vi "pco.labview_Example.vi"() -> ()   [LabVIEW 2020]
uses:
  CameraAccess.lvlib
  Structures.lvlib
  RecordingControl.lvlib
  ImageSensor.lvlib
  GeneralCameraControl.lvlib
  Recorder.lvlib
  TimingControl.lvlib
panel:
  out "exposureMinLimit":u64
  out "exposureMaxLimit":u64
  out "strSensor":T1
  in  "wRegionType":u16(ring) items=["REGION_TYPE_BALANCED", "REGION_TYPE_CENTER_BASED", "REGION_TYPE_CORNER_BASED", "REGION_TYPE_FULL", "REGION_TYPE_CUSTOM"]
  in  "wExpBase":u16(ring)=2 items=["ns", "us", "ms"]
  in  "dwMinExposure":u32=1 min=1 step=1
  in  "dwMaxExposure":u32=100 min=1 step=1
  in  "wSmoothness":u16=1 caption="Smoothness" min=1 max=10 step=1
  in  "bAutoExp":bool caption="Auto Exp On"
  in  "wRamSegment":u16[](array[numeric]) caption="Ram Segment\n(only CamRam)"
  in  "Get Image":bool
  out "bFIFOOverflow":bool[](array[boolean]) caption="FIFO Overflow"
  in  "Init":bool
  in  "baseName":string caption="Base File Name \n(only file, not mandatory)"
  in  "ResetRecorder":bool caption="Stop Copy"
  out "Image":u16[][](graph)
  in  "Quit":bool
  in  "Stop recording":bool
  in  "Start recording":bool
  in  "Create":bool
  in  "roiY1":u16=2 min=2 max=5120 step=1
  in  "roiX1":u16=2 min=2 max=896 step=1
  in  "roiY0":u16=1 min=1 max=5119 step=1
  in  "roiX0":u16=1 min=1 max=895 step=1
  out "Image Height":u16
  out "Image Width":u16
  in  "Image Index":u32 max=9
  in  "Cam Index":u32 max=0 step=1
  out "dwReqImgCount":u32[](array[numeric]) caption="Required Number of Images (Indicator)"
  out "stopTime[ms]":u32[](array[numeric]) caption="Stop Time  of Record [ms]"
  out "bBuffersFull":bool[](array[boolean]) caption="ReqImg Recorded"
  out "dwProcImgCount":u32[](array[numeric]) caption="Currently Recorded Images"
  out "lastError":u32[](array[numeric]) caption="Last Error" format="%x"
  out "bIsRunning":bool[](array[boolean]) caption="Acquiring Flag"
  out "startTime[ms]":u32[](array[numeric]) caption="Start Time  of Record [ms]"
  in  "dwImgCountArr":u32[](array[numeric]) caption="Required Number \nof Images" min=4
  out "phRec":u64
  out "dwMaxImgCountArr":u32[](array[numeric]) caption="Max Number of Recordable Images"
  in  "dwImgDistributionArr":u32[](array[numeric]) caption="Memory Distribution" min=1
  in  "szPath":path=path "C:/" caption="Destination Folder"
  in  "wType":u16(ring)=1 caption="Type" items=["PCO_RECORDER_MEMORY_SEQUENCE"=1, "PCO_RECORDER_MEMORY_RINGBUF"=2, "PCO_RECORDER_MEMORY_FIFO"=3]
  in  "dwRecMode":u16(ring)=1 caption="Recorder Mode" items=["PCO_RECORDER_MODE_FILE"=1, "PCO_RECORDER_MODE_MEMORY"=2, "PCO_RECORDER_MODE_CAMRAM"=3]
  out "Error":errorcluster {"code" format="%x"}
  out "phCam":u64[](array[numeric])
  # "This is the main example program showing the different possibilities of recording images with pco cameras\nThe usage is guided by disabling/enabling the required parts of the front panel.\nLive images are shown during record\nImages can be read after acquisition is finished/stopped\nFor detailed information watch the Use_pco.labview_Example.avi video\n\n+ If you want a example with live stream images, take a look at pco.labview_Live_Example.vi\n+ If you want a small example to start building your own application, you can also use pco.labview_Simple_example.vi"
  # "pco.labview"
  # "Create Parameters"
  # "Auto Exposure"
  # "Init Parameters"
  # "Acquire Images"
  # "Status Indicators"
  # "Parameters for image readout"
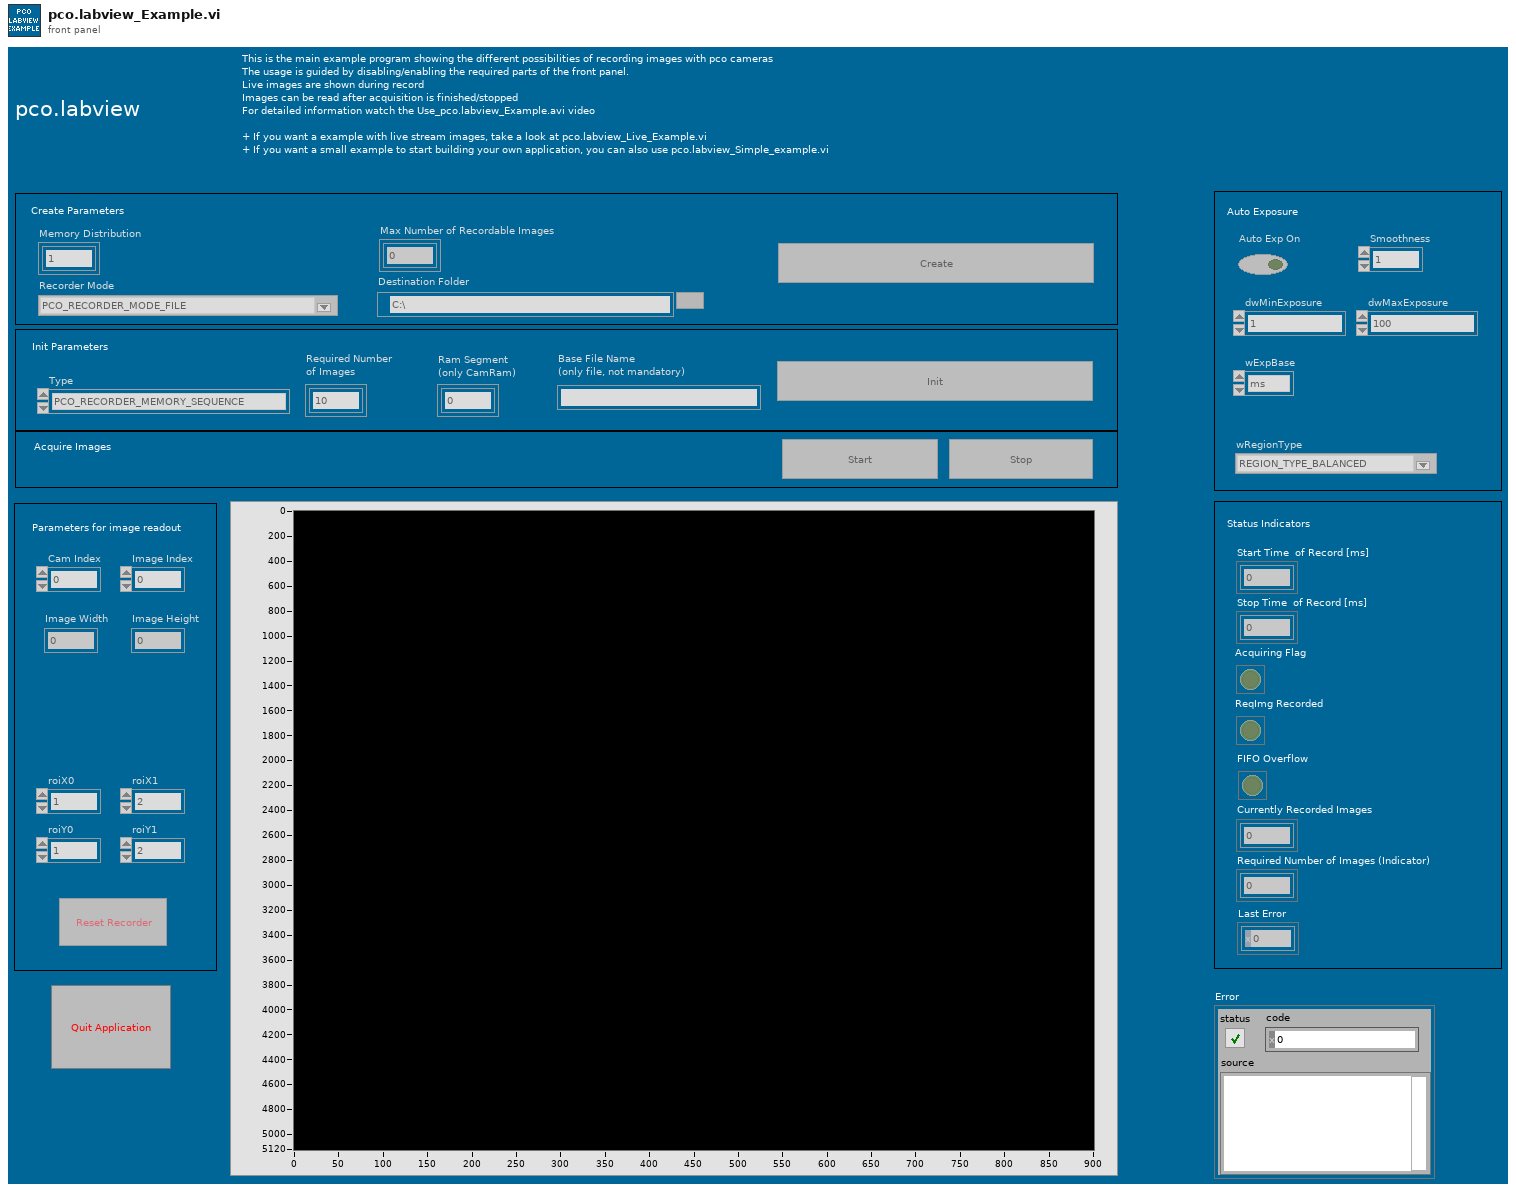
[diagram p1: front panel]
types:
  T1 = cluster{"PCO_Description":cluster{"wSensorTypeDESC":u16, "wSensorSubTypeDESC":u16, "wMaxHorzResStdDESC":u16, "wMaxVertResStdDESC":u16, "wMaxHorzResExtDESC":u16, "wMaxVertResExtDESC":u16, "wDynResDESC":u16, "wMaxBinHorzDESC":u16, "wBinHorzSteppingDESC":u16, "wMaxBinVertDESC":u16, "wBinVertSteppingDESC":u16, "wRoiHorStepsDESC":u16, "wRoiVertStepsDESC":u16, "wNumADCsDESC":u16, "wMinSizeHorzDESC":u16, "dwPixelRateDESC":u32[], "wConvFactDESC":u16[], "sCoolingSetpoints":i16[], "wSoftRoiHorStepsDESC":u16, "wSoftRoiVertStepsDESC":u16, "wIRDESC":u16, "wMinSizeVertDESC":u16, "dwMinDelayDESC":u32, "dwMaxDelayDESC":u32, "dwMinDelayStepDESC":u32, "dwMinExposureDESC":u32, "dwMaxExposureDESC":u32, "dwMinExposureStepDESC":u32, "dwMinDelayIRDESC":u32, "dwMaxDelayIRDESC":u32, "dwMinExposureIRDESC":u32, "dwMaxExposureIRDESC":u32, "wTimeTableDESC":u16, "wDoubleImageDESC":u16, "sMinCoolSetDESC":i16, "sMaxCoolSetDESC":i16, "sDefaultCoolSetDESC":i16, "wPowerDownModeDESC":u16, "wOffsetRegulationDESC":u16, "wColorPatternDESC":u16, "wPatternTypeDESC":u16, "wNumCoolingSetpoints":u16, "dwGeneralCapsDESC1":u32, "dwGeneralCapsDESC2":u32, "dwExtSyncFrequency":u32[], "dwGeneralCapsDESC3":u32, "dwGeneralCapsDESC4":u32}, "PCO_Description2":cluster{"dwMinPeriodicalTimeDESC2":u32, "dwMaxPeriodicalTimeDESC2":u32, "dwMinPeriodicalConditionDESC2":u32, "dwMaxNumberOfExposuresDESC2":u32, "lMinMonitorSignalOffsetDESC2":i32, "dwMaxMonitorSignalOffsetDESC2":u32, "dwMinPeriodicalStepDESC2":u32, "dwStartTimeDelayDESC2":u32, "dwMinMonitorStepDESC2":u32, "dwMinDelayModDESC2":u32, "dwMaxDelayModDESC2":u32, "dwMinDelayStepModDESC2":u32, "dwMinExposureModDESC2":u32, "dwMaxExposureModDESC2":u32, "dwMinExposureStepModDESC2":u32, "dwModulateCapsDESC2":u32}, "PCO_Description_Intensified":cluster{"wChannelNumberIntensifiedDESC":u16, "wNumberOfChannelsIntensifiedDESC":u16, "wMinVoltageIntensifiedDESC":u16, "wMaxVoltageIntensifiedDESC":u16, "wVoltageStepIntensifiedDESC":u16, "wExtendedMinVoltageIntensifiedDESC":u16, "wMaxLoopCountIntensifiedDESC":u16, "dwMinPhosphorDecayIntensified_ns_DESC":u32, "dwMaxPhosphorDecayIntensified_ms_DESC":u32, "dwFlagsIntensifiedDESC":u32, "szIntensifierTypeDESC":string, "dwMCP_RectangleXL_DESC":u32, "dwMCP_RectangleXR_DESC":u32, "dwMCP_RectangleYT_DESC":u32, "dwMCP_RectangleYB_DESC":u32}, "PCO_Description3":cluster{"wDarkOffsetDESC3":u16, "dwGeneralCapsDESC3_1":u32, "dwGeneralCapsDESC3_2":u32, "dwGeneralCapsDESC3_3":u32, "dwGeneralCapsDESC3_4":u32, "wMinHorzResStdDESC3":u16, "wMinVertResStdDESC3":u16, "wMinHorzResExtDESC3":u16, "wMinVertResExtDESC3":u16, "dPixelsize_horzDESC3_um":dbl, "dPixelsize_vertDESC3_um":dbl, "dMinSensorTempWarningDESC3_C":dbl, "dMaxSensorTempWarningDESC3_C":dbl, "dMinCameraTempWarningDESC3_C":dbl, "dMaxCameraTempWarningDESC3_C":dbl, "dMinPowerTempWarningDESC3_C":dbl, "dMaxPowerTempWarningDESC3_C":dbl, "dMinPowerVoltageWarningDESC3_V":dbl, "dMaxPowerVoltageWarningDESC3_V":dbl, "dMinSensorTempErrorDESC3_C":dbl, "dMaxSensorTempErrorDESC3_C":dbl, "dMinCameraTempErrorDESC3_C":dbl, "dMaxCameraTempErrorDESC3_C":dbl, "dMinPowerTempErrorDESC3_C":dbl, "dMaxPowerTempErrorDESC3_C":dbl, "dMinPowerVoltageErrorDESC3_V":dbl, "dMaxPowerVoltageErrorDESC3_V":dbl}, "wSensorformat":u16, "wRoiX0":u16, "wRoiY0":u16, "wRoiX1":u16, "wRoiY1":u16, "wBinHorz":u16, "wBinVert":u16, "wIntensifiedFlags":u16, "dwPixelRate":u32, "wConvFact":u16, "wDoubleImage":u16, "wADCOperation":u16, "wIR":u16, "sCoolSet":i16, "wOffsetRegulation":u16, "wNoiseFilterMode":u16, "wFastReadoutMode":u16, "wDSNUAdjustMode":u16, "wCDIMode":u16, "wIntensifiedVoltage":u16, "wIntensifiedGatingMode":u16, "dwIntensifiedPhosphorDecay_us":u32, "PCO_Signal_Description":cluster{"wNumOfSignals":u16, "strSingeSignalDesc":cluster{"strSignalName":string[], "wSignalDefinitions":u16, "wSignalTypes":u16, "wSignalPolarity":u16, "wSignalFilter":u16}[]}}
  T2 = enum8{"Enabled", "Disabled", "Disabled and Grayed Out"}
  T3 = cluster{"wInterfaceType":u16, "wCameraNumber":u16, "wCameraNumAtInterface":u16, "wOpenFlags":u16[], "dwOpenFlags":u32[], "wOpenPtr":u64[]}
  T4 = cluster{"wSensorTypeDESC":u16, "wSensorSubTypeDESC":u16, "wMaxHorzResStdDESC":u16, "wMaxVertResStdDESC":u16, "wMaxHorzResExtDESC":u16, "wMaxVertResExtDESC":u16, "wDynResDESC":u16, "wMaxBinHorzDESC":u16, "wBinHorzSteppingDESC":u16, "wMaxBinVertDESC":u16, "wBinVertSteppingDESC":u16, "wRoiHorStepsDESC":u16, "wRoiVertStepsDESC":u16, "wNumADCsDESC":u16, "wMinSizeHorzDESC":u16, "dwPixelRateDESC":u32[], "wConvFactDESC":u16[], "sCoolingSetpoints":i16[], "wSoftRoiHorStepsDESC":u16, "wSoftRoiVertStepsDESC":u16, "wIRDESC":u16, "wMinSizeVertDESC":u16, "dwMinDelayDESC":u32, "dwMaxDelayDESC":u32, "dwMinDelayStepDESC":u32, "dwMinExposureDESC":u32, "dwMaxExposureDESC":u32, "dwMinExposureStepDESC":u32, "dwMinDelayIRDESC":u32, "dwMaxDelayIRDESC":u32, "dwMinExposureIRDESC":u32, "dwMaxExposureIRDESC":u32, "wTimeTableDESC":u16, "wDoubleImageDESC":u16, "sMinCoolSetDESC":i16, "sMaxCoolSetDESC":i16, "sDefaultCoolSetDESC":i16, "wPowerDownModeDESC":u16, "wOffsetRegulationDESC":u16, "wColorPatternDESC":u16, "wPatternTypeDESC":u16, "wNumCoolingSetpoints":u16, "dwGeneralCapsDESC1":u32, "dwGeneralCapsDESC2":u32, "dwExtSyncFrequency":u32[], "dwGeneralCapsDESC3":u32, "dwGeneralCapsDESC4":u32}
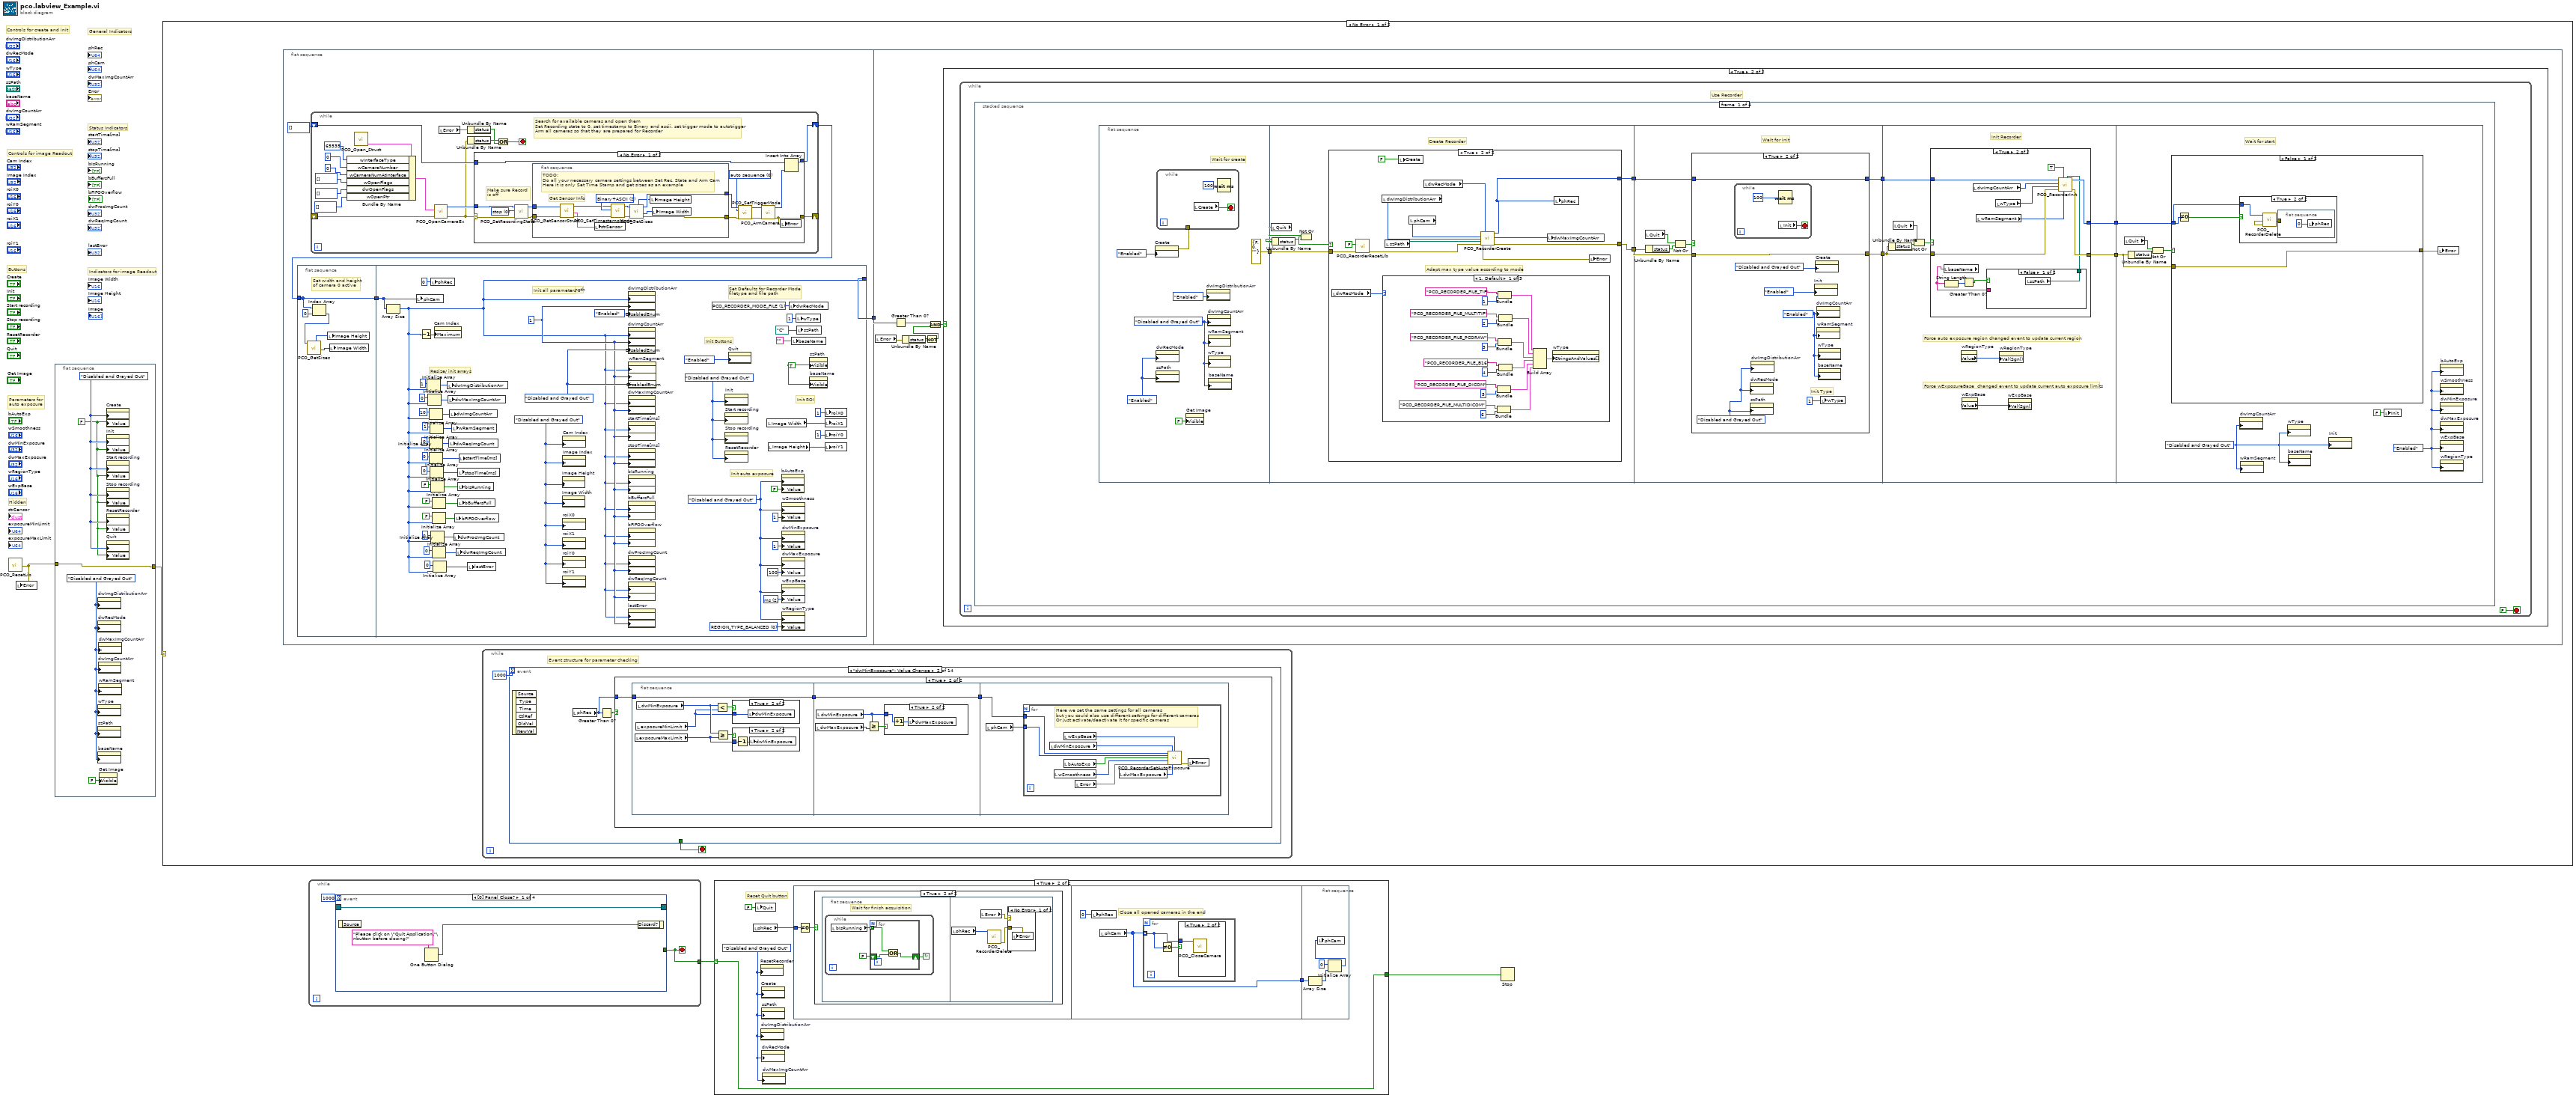
[diagram p0: block diagram]
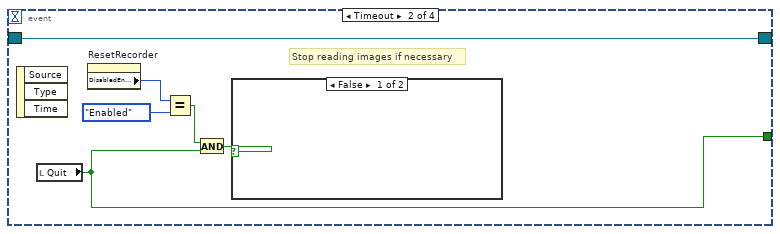
[diagram p6: hidden frame]
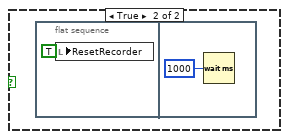
[diagram p7: hidden frame]
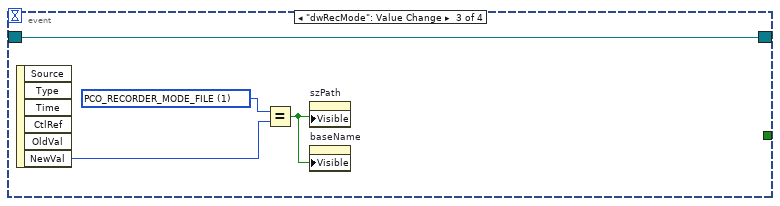
[diagram p8: hidden frame]
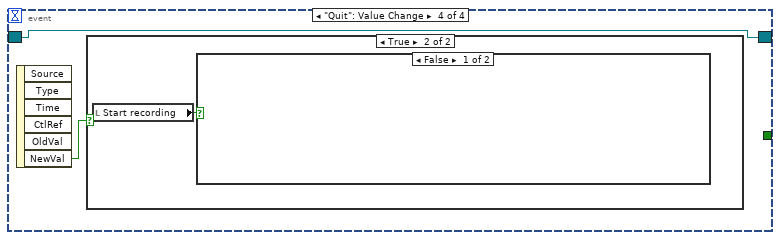
[diagram p9: hidden frame]
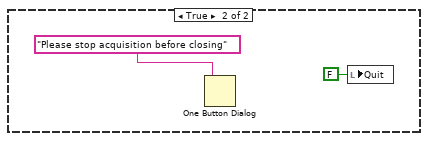
[diagram p11: hidden frame]
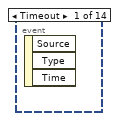
[diagram p12: hidden frame]
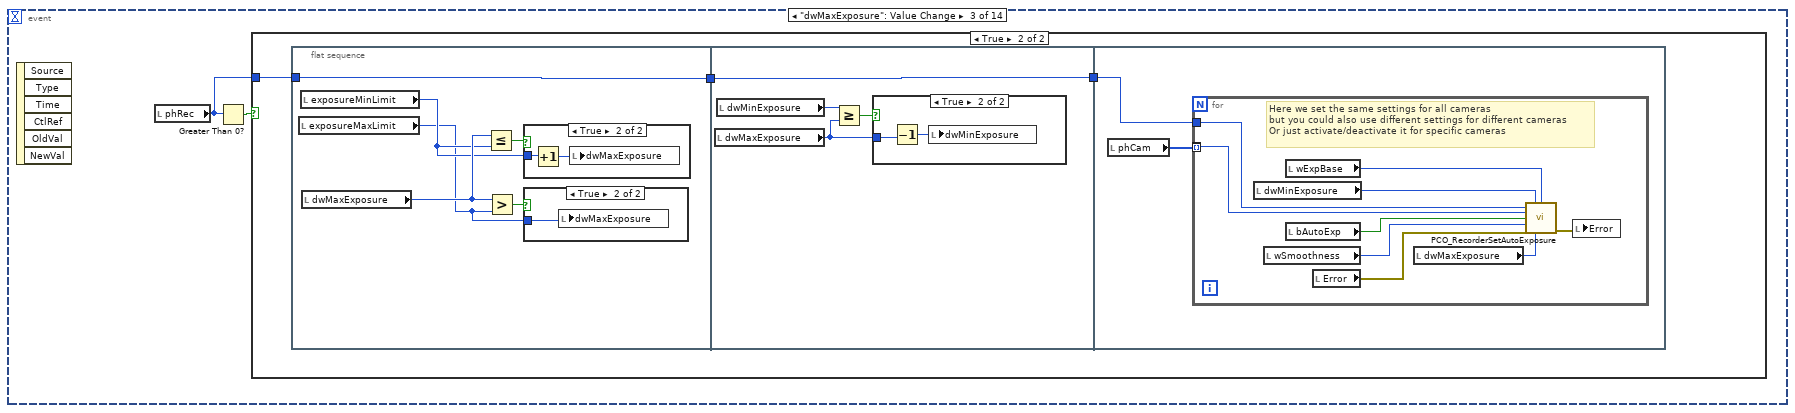
[diagram p17: hidden frame]
diagram:
  # "Hidden"
  # "Parameters for \nauto exposure"
  # "Buttons"
  # "Indicators for image Readout"
  # "Controls for image Readout"
  # "Status Indicators"
  # "Controls for create and init"
  # "General Indicators"
  n1 = call "PCO_ResetLib.vi"() -> ("error out"=w3:errorcluster)  [unwired: 10 in, 1 out]
  n2 = local write "Error"(w3) -> ()
  n3 = flat-sequence {
    tunnel: w3 -> [w9]
    tunnel: [w9] -> w2
    frame #0 {
      w5 = T2."Disabled and Grayed Out" ("Disabled")
      w7 = FALSE
      w8 = T2."Disabled and Grayed Out" ("Disabled")
      n4 = property on="dwImgDistributionArr" class="Arr (strict)"("DisabledEnum"=w5) -> ()  [unwired: 2 in, 2 out]
      n5 = property on="dwRecMode" class="Ring (strict)"("DisabledEnum"=w5) -> ()  [unwired: 2 in, 2 out]
      n6 = property on="wType" class="Ring (strict)"("DisabledEnum"=w5) -> ()  [unwired: 2 in, 2 out]
      n7 = property on="szPath" class="Path"("DisabledEnum"=w5) -> ()  [unwired: 2 in, 2 out]
      n8 = property on="baseName" class="Str"("DisabledEnum"=w5) -> ()  [unwired: 2 in, 2 out]
      n9 = property on="dwImgCountArr" class="Arr (strict)"("DisabledEnum"=w5) -> ()  [unwired: 2 in, 2 out]
      n10 = property on="dwMaxImgCountArr" class="Arr (strict)"("DisabledEnum"=w5) -> ()  [unwired: 2 in, 2 out]
      n11 = property on="wRamSegment" class="Arr (strict)"("DisabledEnum"=w5) -> ()  [unwired: 2 in, 2 out]
      n12 = property on="Get Image" class="Bool (strict)"("Visible"=FALSE) -> ()  [unwired: 2 in, 2 out]
      n13 = property on="Create" class="Bool (strict)"("DisabledEnum"=w8, "Value"=w7) -> ()  [unwired: 2 in, 2 out]
      n14 = property on="Init" class="Bool (strict)"("DisabledEnum"=w8, "Value"=w7) -> ()  [unwired: 2 in, 2 out]
      n15 = property on="Start recording" class="Bool (strict)"("DisabledEnum"=w8, "Value"=w7) -> ()  [unwired: 2 in, 2 out]
      n16 = property on="Stop recording" class="Bool (strict)"("DisabledEnum"=w8, "Value"=w7) -> ()  [unwired: 2 in, 2 out]
      n17 = property on="ResetRecorder" class="Bool (strict)"("DisabledEnum"=w8, "Value"=w7) -> ()  [unwired: 2 in, 2 out]
      n18 = property on="Quit" class="Bool (strict)"("DisabledEnum"=w8, "Value"=w7) -> ()  [unwired: 2 in, 2 out]
    }
  }
  n19 = case shown="No Error" w2 {
    frame No Error {
      n20 = flat-sequence {
        tunnel: [w203] -> w10
        tunnel: w10 -> [w307]
        frame #0 {
          n21 = flat-sequence {
            tunnel: w202 -> [w208]
            tunnel: [w208] -> w201
            tunnel: [w217] -> w203
            tunnel: w201 -> [w219]
            frame #0 {
              # "Set width and height\nof camera 0 active"
              n22 = Index Array(array=w208, index=0) -> (element=w205:u64)
              n23 = call "PCO_GetSizes.vi"("ph"=w205) -> ("wXResAct"=w207:u16, "wYResAct"=w206:u16)  [unwired: 4 in, 5 out]
              n24 = local write "Image Height"(w206) -> ()
              n25 = local write "Image Width"(w207) -> ()
            }
            frame #1 {
              w210 = u16 0 items=["REGION_TYPE_BALANCED", "REGION_TYPE_CENTER_BASED", "REGION_TYPE_CORNER_BASED", "REGION_TYPE_FULL", "REGION_TYPE_CUSTOM"] ("wRegionType")
              w211 = u16 2 items=["ns", "us", "ms"] ("wExpBase")
              w216 = u16 1 items=["PCO_RECORDER_MODE_FILE"=1, "PCO_RECORDER_MODE_MEMORY"=2, "PCO_RECORDER_MODE_CAMRAM"=3] ("dwRecMode")
              w221 = T2."Disabled and Grayed Out" ("Disabled")
              w226 = T2."Disabled and Grayed Out" ("Disabled")
              w230 = T2."Disabled and Grayed Out" ("Disabled")
              w237 = TRUE
              w225 = T2."Disabled and Grayed Out" ("Disabled")
              w224 = u32 1 ("Number of Rows")
              # "Init auto exposure"
              # "Init Buttons"
              # "Init ROI"
              # "Set Defaults for Recorder Mode\nfiletype and file path"
              # "Set Fixed array length"
              # "Resize/ init arrays"
              # "Init all parameters"
              n26 = Array Size(array=w219) -> (size(s)=w217:i32)
              n27 = local write "phCam"(w219) -> ()
              n28 = Decrement(x=w217) -> (x-1=w218:i32)
              n29 = Initialize Array(u32 1 ("element"), w217) -> (w260:u32[])
              n30 = Initialize Array(u32 0 ("element"), w217) -> (w258:u32[])
              n31 = Initialize Array(u32 10 ("element"), w217) -> (w240:u32[])
              n32 = Initialize Array(u32 0 ("element"), w217) -> (w255:u32[])
              n33 = Initialize Array(u32 0 ("element"), w217) -> (w249:u32[])
              n34 = Initialize Array(u16 1 ("element"), w217) -> (w222:u16[])
              n35 = Initialize Array(u32 0 ("element"), w217) -> (w251:u32[])
              n36 = local write "phRec"(u64 0 ("phRec")) -> ()
              n37 = Initialize Array(u32 0 ("element"), w217) -> (w246:u32[])
              n38 = Initialize Array(FALSE, w217) -> (w254:bool[])
              n39 = Initialize Array(FALSE, w217) -> (w247:bool[])
              n40 = Initialize Array(FALSE, w217) -> (w227:bool[])
              n41 = Initialize Array(u32 0 ("element"), w217) -> (w243:u32[])
              n42 = Initialize Array(u32 0 ("element"), w217) -> (w242:u32[])
              n43 = property on="Cam Index" class="DigNum (strict)"("Maximum"=w218) -> ()  [unwired: 2 in, 2 out]
              n44 = local write "dwImgDistributionArr"(w260) -> ()
              n45 = local write "dwMaxImgCountArr"(w258) -> ()
              n46 = local write "dwReqImgCount"(w255) -> ()
              n47 = local write "dwImgCountArr"(w240) -> ()
              n48 = local write "wRamSegment"(w222) -> ()
              n49 = local write "dwProcImgCount"(w246) -> ()
              n50 = local write "bFIFOOverflow"(w227) -> ()
              n51 = local write "dwReqImgCount"(w243) -> ()
              n52 = local write "bIsRunning"(w254) -> ()
              n53 = local write "stopTime[ms]"(w251) -> ()
              n54 = local write "bBuffersFull"(w247) -> ()
              n55 = local write "startTime[ms]"(w249) -> ()
              n56 = local write "lastError"(w242) -> ()
              n57 = property on="Image Height" class="DigNum (strict)"("DisabledEnum"=w226) -> ()  [unwired: 2 in, 2 out]
              n58 = property on="Image Width" class="DigNum (strict)"("DisabledEnum"=w226) -> ()  [unwired: 2 in, 2 out]
              n59 = property on="Cam Index" class="DigNum (strict)"("DisabledEnum"=w226) -> ()  [unwired: 2 in, 2 out]
              n60 = property on="Image Index" class="DigNum (strict)"("DisabledEnum"=w226) -> ()  [unwired: 2 in, 2 out]
              n61 = property on="roiX0" class="DigNum (strict)"("DisabledEnum"=w226) -> ()  [unwired: 2 in, 2 out]
              n62 = property on="roiX1" class="DigNum (strict)"("DisabledEnum"=w226) -> ()  [unwired: 2 in, 2 out]
              n63 = property on="roiY0" class="DigNum (strict)"("DisabledEnum"=w226) -> ()  [unwired: 2 in, 2 out]
              n64 = property on="roiY1" class="DigNum (strict)"("DisabledEnum"=w226) -> ()  [unwired: 2 in, 2 out]
              n65 = property on="dwImgDistributionArr" class="Arr (strict)"("Number of Columns"=w217, "Number of Rows"=w224, "DisabledEnum"=T2."Enabled" ("Disabled")) -> ()  [unwired: 2 in, 2 out]
              n66 = property on="dwImgCountArr" class="Arr (strict)"("Number of Columns"=w217, "Number of Rows"=w224, "DisabledEnum"=w225) -> ()  [unwired: 2 in, 2 out]
              n67 = property on="dwMaxImgCountArr" class="Arr (strict)"("Number of Columns"=w217, "Number of Rows"=w224) -> ()  [unwired: 2 in, 2 out]
              n68 = property on="startTime[ms]" class="Arr (strict)"("Number of Columns"=w217, "Number of Rows"=w224) -> ()  [unwired: 2 in, 2 out]
              n69 = property on="stopTime[ms]" class="Arr (strict)"("Number of Columns"=w217, "Number of Rows"=w224) -> ()  [unwired: 2 in, 2 out]
              n70 = property on="bIsRunning" class="Arr (strict)"("Number of Columns"=w217, "Number of Rows"=w224) -> ()  [unwired: 2 in, 2 out]
              n71 = property on="bBuffersFull" class="Arr (strict)"("Number of Columns"=w217, "Number of Rows"=w224) -> ()  [unwired: 2 in, 2 out]
              n72 = property on="bFIFOOverflow" class="Arr (strict)"("Number of Columns"=w217, "Number of Rows"=w224) -> ()  [unwired: 2 in, 2 out]
              n73 = property on="dwProcImgCount" class="Arr (strict)"("Number of Columns"=w217, "Number of Rows"=w224) -> ()  [unwired: 2 in, 2 out]
              n74 = property on="dwReqImgCount" class="Arr (strict)"("Number of Columns"=w217, "Number of Rows"=w224) -> ()  [unwired: 2 in, 2 out]
              n75 = property on="lastError" class="Arr (strict)"("Number of Columns"=w217, "Number of Rows"=w224) -> ()  [unwired: 2 in, 2 out]
              n76 = property on="wRamSegment" class="Arr (strict)"("Number of Columns"=w217, "Number of Rows"=w224, "DisabledEnum"=w225) -> ()  [unwired: 2 in, 2 out]
              n77 = property on="Init" class="Bool (strict)"("DisabledEnum"=w230) -> ()  [unwired: 2 in, 2 out]
              n78 = property on="Start recording" class="Bool (strict)"("DisabledEnum"=w230) -> ()  [unwired: 2 in, 2 out]
              n79 = property on="Stop recording" class="Bool (strict)"("DisabledEnum"=w230) -> ()  [unwired: 2 in, 2 out]
              n80 = property on="ResetRecorder" class="Bool (strict)"("DisabledEnum"=w230) -> ()  [unwired: 2 in, 2 out]
              n81 = property on="Quit" class="Bool (strict)"("DisabledEnum"=T2."Enabled" ("Disabled")) -> ()  [unwired: 2 in, 2 out]
              n82 = local read "Image Width"() -> (w234:u16)
              n83 = local read "Image Height"() -> (w233:u16)
              n84 = property on="bAutoExp" class="Bool (strict)"("DisabledEnum"=w221, "Value"=FALSE ("bAutoExp")) -> ()  [unwired: 2 in, 2 out]
              n85 = property on="wSmoothness" class="DigNum (strict)"("DisabledEnum"=w221, "Value"=u16 1 ("wSmoothness")) -> ()  [unwired: 2 in, 2 out]
              n86 = property on="dwMinExposure" class="DigNum (strict)"("DisabledEnum"=w221, "Value"=u32 1 ("dwMinExposure")) -> ()  [unwired: 2 in, 2 out]
              n87 = property on="dwMaxExposure" class="DigNum (strict)"("DisabledEnum"=w221, "Value"=u32 100 ("dwMaxExposure")) -> ()  [unwired: 2 in, 2 out]
              n88 = property on="wExpBase" class="Ring (strict)"("DisabledEnum"=w221, "Value"=w211) -> ()  [unwired: 2 in, 2 out]
              n89 = property on="wRegionType" class="Ring (strict)"("DisabledEnum"=w221, "Value"=w210) -> ()  [unwired: 2 in, 2 out]
              n90 = local write "dwRecMode"(w216) -> ()
              n91 = local write "baseName"("" ("szFilePath")) -> ()
              n92 = local write "wType"(u16 1 ("wType")) -> ()
              n93 = local write "szPath"(path "C:/" ("szFilePath")) -> ()
              n94 = property on="szPath" class="Path"("Visible"=w237) -> ()  [unwired: 2 in, 2 out]
              n95 = property on="baseName" class="Str"("Visible"=w237) -> ()  [unwired: 2 in, 2 out]
              n96 = local write "roiX0"(u16 1 ("roiX0")) -> ()
              n97 = local write "roiX1"(w234) -> ()
              n98 = local write "roiY0"(u16 1 ("roiY0")) -> ()
              n99 = local write "roiY1"(w233) -> ()
            }
          }
          n100 = while {
            shift-right: [w277] -> w202
            shift-left: u64[] [] -> [w276]
            shift-right: [w275] -> _
            shift-left: _ -> [w279]
            stop <- w271 stop-if-true
            # "Search for available cameras and open them\nSet Recording state to 0, set timestamp to Binary and ascii, set trigger mode to autotrigger\nArm all cameras so that they are prepared for Recorder"
            n101 = call "PCO_Open_Struct.vi"() -> ("PCO_Open_Struct"=w269:T3)  [unwired: 4 in, 4 out]
            n102 = Bundle By Name(cluster=w269, "wInterfaceType"=u16 65535, "wCameraNumber"=u16 0, "wCameraNumAtInterface"=u16 0, "wOpenFlags"=u16[] [], "dwOpenFlags"=u32[] [], "wOpenPtr"=u64[] []) -> (w262:T3)
            n103 = call "PCO_OpenCameraEx.vi"("error in (no error)"=w279, "strOpenStruct"=w262) -> ("error out"=w270:errorcluster, "ph out"=w278:u64)  [unwired: 7 in, 1 out]
            n104 = local read "Error"() -> (w274:errorcluster)
            n105 = Unbundle By Name(w274) -> ("status"=w272:bool)
            n106 = Unbundle By Name(w270) -> ("status"=w273:bool)
            n107 = case shown="No Error" w270 {
              selector: w270 -> [w289 _]
              tunnel: w278 -> [w290 _]
              tunnel: [w291 errorcluster {"status"=FALSE, "code"=0, "source"=""} ("error out")] -> w275
              tunnel: w276 -> [w286 w306]
              tunnel: [w287 w306] -> w277
              frame No Error {
                w280 = u16 0 items=["auto sequence"=0, "software trigger"=1, "external exposure start & software trigger"=2, "external exposure control"=3, "external synchronized"=4, "fast external exposure control"=5, "external CDS control"=6, "slow external exposure control"=7, "external synchronized HDSDI"=258] ("wTriggerMode")
                w288 = u16 0 items=["stop", "run"] ("wRecState")
                # "Make sure Record \nis off"
                n108 = call "PCO_SetRecordingState.vi"("error in (no error)"=w289, "wRecState"=w288, "ph"=w290) -> ("error out"=w293:errorcluster, "ph out"=w292:u64)  [unwired: 6 in, 1 out]
                n109 = flat-sequence {
                  tunnel: w293 -> [w304]
                  tunnel: w292 -> [w296]
                  tunnel: [w300] -> w283
                  tunnel: [w301] -> w284
                  frame #0 {
                    w298 = u16 2 items=["OFF", "Binary", "Binary+ASCII", "ASCII"] ("wTimeStampMode")
                    # "Get Sensor Info"
                    # "TODO:\nDo all your necessary camera settings between Set Rec. State and Arm Cam\nHere it is only Set Time Stamp and get sizes as an example"
                    n110 = call "PCO_GetSensorStruct.vi"("ph"=w296) -> ("strSensor"=w294:T1, "ph out"=w295:u64)  [unwired: 6 in, 2 out]
                    n111 = local write "strSensor"(w294) -> ()
                    n112 = call "PCO_SetTimestampMode.vi"("error in (no error)"=w304, "wTimeStampMode"=w298, "ph"=w295) -> ("error out"=w303:errorcluster, "ph out"=w302:u64)  [unwired: 6 in, 1 out]
                    n113 = call "PCO_GetSizes.vi"("error in (no error)"=w303, "ph"=w302) -> ("error out"=w300:errorcluster, "wXResAct"=w297:u16, "ph out"=w301:u64, "wYResAct"=w299:u16)  [unwired: 3 in, 3 out]
                    n114 = local write "Image Height"(w299) -> ()
                    n115 = local write "Image Width"(w297) -> ()
                  }
                }
                n116 = call "PCO_SetTriggerMode.vi"("error in (no error)"=w283, "wTriggerMode"=w280, "ph"=w284) -> ("error out"=w282:errorcluster, "ph out"=w281:u64)  [unwired: 6 in, 1 out]
                n117 = call "PCO_ArmCamera.vi"("error in (no error)"=w282, "ph"=w281) -> ("error out"=w291:errorcluster, "ph out"=w285:u64)  [unwired: 7 in, 1 out]
                n118 = local write "Error"(w291) -> ()
                n119 = Insert Into Array(array=w286, new element=w285) -> (w287:u64[])  [unwired: 1 in]
              }
              frame Error {
              }
            }
            n120 = Or(x=w273, y=w272) -> (x .or. y?=w271:bool)
          }
        }
        frame #1 {
          n121 = local read "Error"() -> (w312:errorcluster)
          n122 = Greater Than 0?(x=w307) -> (x > 0?=w311:bool)
          n123 = Unbundle By Name(w312) -> ("status"=w309:bool)
          n124 = Not(x=w309) -> (.not. x?=w308:bool)
          n125 = And(x=w311, y=w308) -> (x .and. y?=w310:bool)
          n126 = case shown="True" w310 {
            frame False {
              n127 = property on="Create" class="Bool (strict)"("DisabledEnum"=T2."Disabled and Grayed Out" ("Disabled")) -> ()  [unwired: 2 in, 2 out]
              n128 = One Button Dialog(message="No cameras found for recorder\nPlease stop application, switch on your camera(s) and try again") -> ()  [unwired: 1 in, 1 out]
            }
            frame True {
              n129 = while {
                stop <- FALSE stop-if-true
                # "Use Recorder"
                n130 = stacked-sequence {
                  frame #0 {
                    n131 = flat-sequence {
                      tunnel: [errorcluster {"status"=FALSE, "code"=0, "source"=""} ("Error")] -> w319
                      tunnel: [w337] -> w322
                      tunnel: w319 -> [w334]
                      tunnel: [w332] -> w318
                      tunnel: w322 -> [w395]
                      tunnel: [w394] -> w321
                      tunnel: w318 -> [w393]
                      tunnel: [w392] -> w317
                      tunnel: w321 -> [w415]
                      tunnel: [w414] -> w320
                      tunnel: w317 -> [w412]
                      tunnel: [w409] -> w316
                      tunnel: w320 -> [w442]
                      tunnel: w316 -> [w436]
                      frame #0 {
                        w326 = T2."Enabled" ("Disabled")
                        w324 = T2."Disabled and Grayed Out" ("Disabled")
                        # "Wait for create"
                        n132 = property on="Create" class="Bool (strict)"("DisabledEnum"=T2."Enabled" ("Disabled")) -> (error out=w323:errorcluster)  [unwired: 2 in, 1 out]
                        n133 = property on="dwRecMode" class="Ring (strict)"("DisabledEnum"=w326) -> ()  [unwired: 2 in, 2 out]
                        n134 = property on="szPath" class="Path"("DisabledEnum"=w326) -> ()  [unwired: 2 in, 2 out]
                        n135 = while {
                          tunnel: w323 -> [_]
                          stop <- w330 stop-if-true
                          n136 = local read "Create"() -> (w330:bool)
                          n137 = Wait (ms)(milliseconds to wait=u32 100) -> ()  [unwired: 1 out]
                        }
                        n138 = property on="Get Image" class="Bool (strict)"("Visible"=FALSE) -> ()  [unwired: 2 in, 2 out]
                        n139 = property on="dwImgDistributionArr" class="Arr (strict)"("DisabledEnum"=T2."Enabled" ("Disabled")) -> ()  [unwired: 2 in, 2 out]
                        n140 = property on="dwImgCountArr" class="Arr (strict)"("DisabledEnum"=w324) -> ()  [unwired: 2 in, 2 out]
                        n141 = property on="wRamSegment" class="Arr (strict)"("DisabledEnum"=w324) -> ()  [unwired: 2 in, 2 out]
                        n142 = property on="wType" class="Ring (strict)"("DisabledEnum"=w324) -> ()  [unwired: 2 in, 2 out]
                        n143 = property on="baseName" class="Str"("DisabledEnum"=w324) -> ()  [unwired: 2 in, 2 out]
                      }
                      frame #1 {
                        # "Create Recorder"
                        n144 = local read "Quit"() -> (w335:bool)
                        n145 = Unbundle By Name(w334) -> ("status"=w333:bool)
                        n146 = Not Or(1:w333, 2:w335) -> (0:w336:bool)
                        n147 = case shown="True" w336 {
                          tunnel: [w338 w348] -> w332
                          tunnel: [u64 0 ("phRec out") w346] -> w337
                          tunnel: w334 -> [w338 w343]
                          frame False {
                            # "Wait for finish"
                            n148 = Wait (ms)(milliseconds to wait=u32 100) -> ()  [unwired: 1 out]
                          }
                          frame True {
                            # "Adapt max type value according to mode"
                            n149 = local read "dwRecMode"() -> (w341:u16)
                            n150 = call "PCO_RecorderResetLib.vi"("error in (no error)"=w343, "bSilent"=FALSE) -> ("error out"=w342:errorcluster)  [unwired: 8 in, 1 out]
                            n151 = local read "dwImgDistributionArr"() -> (w351:u32[])
                            n152 = case shown="1, Default" w341 {
                              frame 1, Default {
                                n153 = Bundle("PCO_RECORDER_FILE_MULTIDICOM", u16 6) -> (w353:cluster{string, u16})  [unwired: 1 in]
                                n154 = Bundle("PCO_RECORDER_FILE_DICOM", u16 5) -> (w354:cluster{string, u16})  [unwired: 1 in]
                                n155 = Bundle("PCO_RECORDER_FILE_TIF", u16 1) -> (w371:cluster{string, u16})  [unwired: 1 in]
                                n156 = Bundle("PCO_RECORDER_FILE_PCORAW", u16 3) -> (w360:cluster{string, u16})  [unwired: 1 in]
                                n157 = Bundle("PCO_RECORDER_FILE_MULTITIF", u16 2) -> (w370:cluster{string, u16})  [unwired: 1 in]
                                n158 = Bundle("PCO_RECORDER_FILE_B16", u16 4) -> (w359:cluster{string, u16})  [unwired: 1 in]
                                n159 = Build Array(w371, w370, w360, w359, w354, w353) -> (w369:cluster{string, u16}[])
                                n160 = property on="wType" class="Ring (strict)"("StringsAndValues[]"=w369) -> ()  [unwired: 2 in, 2 out]
                              }
                              frame 2 {
                                n161 = Bundle("PCO_RECORDER_MEMORY_SEQUENCE", u16 1) -> (w381:cluster{string, u16})  [unwired: 1 in]
                                n162 = Bundle("PCO_RECORDER_MEMORY_FIFO", u16 3) -> (w373:cluster{string, u16})  [unwired: 1 in]
                                n163 = Bundle("PCO_RECORDER_MEMORY_RINGBUF", u16 2) -> (w380:cluster{string, u16})  [unwired: 1 in]
                                n164 = Build Array(w381, w380, w373) -> (w379:cluster{string, u16}[])
                                n165 = property on="wType" class="Ring (strict)"("StringsAndValues[]"=w379) -> ()  [unwired: 2 in, 2 out]
                              }
                              frame 3 {
                                n166 = Bundle("PCO_RECORDER_CAMRAM_SEQUENTIAL", u16 1) -> (w388:cluster{string, u16})  [unwired: 1 in]
                                n167 = Bundle("PCO_RECORDER_CAMRAM_SINGLE_IMAGE", u16 2) -> (w387:cluster{string, u16})  [unwired: 1 in]
                                n168 = Build Array(w388, w387) -> (w386:cluster{string, u16}[])
                                n169 = property on="wType" class="Ring (strict)"("StringsAndValues[]"=w386) -> ()  [unwired: 2 in, 2 out]
                              }
                            }
                            n170 = local read "szPath"() -> (w347:path)
                            n171 = local write "Create"(FALSE ("Create and init")) -> ()
                            n172 = local read "phCam"() -> (w352:u64[])
                            n173 = local read "dwRecMode"() -> (w350:u16)
                            n174 = call "PCO_RecorderCreate.vi"("wRecMode"=w350, "phCamArr"=w352, "dwImgDistributionArr"=w351, "szDrive"=w347, "error in (no error)"=w342) -> ("phRec out"=w346:u64, "dwMaxImgCountArr"=w345:u32[], "error out"=w348:errorcluster)  [unwired: 7 in, 1 out]
                            n175 = local write "dwMaxImgCountArr"(w345) -> ()
                            n176 = local write "phRec"(w346) -> ()
                            n177 = local write "Error"(w348) -> ()
                          }
                        }
                      }
                      frame #2 {
                        # "Wait for init"
                        n178 = local read "Quit"() -> (w390:bool)
                        n179 = Unbundle By Name(w393) -> ("status"=w391:bool)
                        n180 = Not Or(1:w391, 2:w390) -> (0:w389:bool)
                        n181 = case shown="True" w389 {
                          tunnel: w395 -> [w397 w402]
                          tunnel: [w397 w402] -> w394
                          tunnel: [w396 w401] -> w392
                          tunnel: w393 -> [w396 w401]
                          frame False {
                          }
                          frame True {
                            w399 = T2."Disabled and Grayed Out" ("Disabled")
                            w400 = T2."Enabled" ("Disabled")
                            # "Init Type"
                            n182 = while {
                              stop <- w406 stop-if-true
                              n183 = Wait (ms)(milliseconds to wait=u32 100) -> ()  [unwired: 1 out]
                              n184 = local read "Init"() -> (w406:bool)
                            }
                            n185 = property on="dwRecMode" class="Ring (strict)"("DisabledEnum"=w399) -> ()  [unwired: 2 in, 2 out]
                            n186 = property on="szPath" class="Path"("DisabledEnum"=w399) -> ()  [unwired: 2 in, 2 out]
                            n187 = property on="dwImgDistributionArr" class="Arr (strict)"("DisabledEnum"=w399) -> ()  [unwired: 2 in, 2 out]
                            n188 = property on="Init" class="Bool (strict)"("DisabledEnum"=T2."Enabled" ("Disabled")) -> ()  [unwired: 2 in, 2 out]
                            n189 = property on="Create" class="Bool (strict)"("DisabledEnum"=T2."Disabled and Grayed Out" ("Disabled")) -> ()  [unwired: 2 in, 2 out]
                            n190 = property on="dwImgCountArr" class="Arr (strict)"("DisabledEnum"=w400) -> ()  [unwired: 2 in, 2 out]
                            n191 = property on="wRamSegment" class="Arr (strict)"("DisabledEnum"=w400) -> ()  [unwired: 2 in, 2 out]
                            n192 = property on="wType" class="Ring (strict)"("DisabledEnum"=w400) -> ()  [unwired: 2 in, 2 out]
                            n193 = property on="baseName" class="Str"("DisabledEnum"=w400) -> ()  [unwired: 2 in, 2 out]
                            n194 = local write "wType"(u16 1) -> ()
                          }
                        }
                      }
                      frame #3 {
                        # "Force wExposureBase  changed event to update current auto exposure limits"
                        # "Force auto exposure region changed event to update current region"
                        # "Init Recorder"
                        n195 = Unbundle By Name(w412) -> ("status"=w411:bool)
                        n196 = local read "Quit"() -> (w410:bool)
                        n197 = Not Or(1:w411, 2:w410) -> (0:w413:bool)
                        n198 = case shown="True" w413 {
                          tunnel: w415 -> [w417 w429]
                          tunnel: [w417 w428] -> w414
                          tunnel: [w416 w427] -> w409
                          tunnel: w412 -> [w416 w426]
                          frame False {
                          }
                          frame True {
                            n199 = local read "baseName"() -> (w425:string)
                            n200 = String Length(string=w425) -> (length=w423:i32)
                            n201 = Greater Than 0?(x=w423) -> (x > 0?=w424:bool)
                            n202 = local read "dwImgCountArr"() -> (w422:u32[])
                            n203 = local read "wRamSegment"() -> (w418:u16[])
                            n204 = case shown="False" w424 {
                              tunnel: w425 -> [_ w433]
                              tunnel: [w430 w431] -> w420
                              frame False {
                                n205 = local read "szPath"() -> (w430:path)
                              }
                              frame True {
                                n206 = local read "szPath"() -> (w432:path)
                                n207 = Build Path(base path=w432, name or relative path=w433) -> (appended path=w431:path)
                              }
                            }
                            n208 = local read "wType"() -> (w419:u16)
                            n209 = call "PCO_RecorderInit.vi"("szFilePath"=w420, "wRamSegmentArr"=w418, "noOverwrite"=TRUE ("wNoOverwrite"), "error in (no error)"=w426, "wType"=w419, "dwImgCountArr"=w422, "phRec"=w429) -> ("error out"=w427:errorcluster, "phRec out"=w428:u64)  [unwired: 2 in, 1 out]
                          }
                        }
                        n210 = property on="wRegionType" class="Ring (strict)"() -> ("Value"=w408:u16)  [unwired: 2 in, 2 out]
                        n211 = property on="wExpBase" class="Ring (strict)"() -> ("Value"=w407:u16)  [unwired: 2 in, 2 out]
                        n212 = property on="wRegionType" class="Ring (strict)"("Val(Sgnl)"=w408) -> ()  [unwired: 2 in, 2 out]
                        n213 = property on="wExpBase" class="Ring (strict)"("Val(Sgnl)"=w407) -> ()  [unwired: 2 in, 2 out]
                      }
                      frame #4 {
                        w435 = T2."Enabled" ("Disabled")
                        w434 = T2."Disabled and Grayed Out" ("Disabled")
                        # "Wait for start"
                        n214 = local read "Quit"() -> (w437:bool)
                        n215 = Unbundle By Name(w436) -> ("status"=w438:bool)
                        n216 = Not Or(1:w438, 2:w437) -> (0:w439:bool)
                        n217 = case shown="False" w439 {
                          tunnel: w442 -> [w445 w452]
                          tunnel: [w443 w449] -> w441
                          tunnel: w436 -> [w443 w453]
                          frame False {
                            n218 = Not Equal To 0?(x=w445) -> (x != 0?=w444:bool)
                            n219 = case shown="True" w444 {
                              tunnel: w445 -> [_ w447]
                              frame False {
                              }
                              frame True {
                                n220 = call "PCO_RecorderDelete.vi"("phRec"=w447) -> ("error out"=w446:errorcluster)  [unwired: 9 in, 1 out]
                                n221 = flat-sequence {
                                tunnel: w446 -> [_]
                                frame #0 {
                                n222 = local write "phRec"(u64 0 ("phRec")) -> ()
                                }
                                }
                              }
                            }
                          }
                          frame True {
                            n223 = local read "dwRecMode"() -> (w455:u16)
                            n224 = Equal?(x=w455, y=u32 3) -> (x = y?=w454:bool)
                            n225 = case shown="True" w454 {
                              tunnel: w453 -> [w458 w462]
                              tunnel: w452 -> [_ w460]
                              tunnel: [w458 w461] -> w451
                              frame False {
                              }
                              frame True {
                                # "For CamRam mode update\nproc image count"
                                n226 = local read "phCam"() -> (w459:u64[])
                                n227 = for {
                                shift-right: [w469] -> w461
                                shift-left: w462 -> [w470]
                                shift-right: [w468] -> _
                                shift-left: w460 -> [w471]
                                tunnel: w459 -> [w467] mode=indexing
                                i -> [w465]
                                n228 = call "PCO_RecorderGetStatus.vi"("phRec"=w471, "phCam"=w467, "error in (no error)"=w470) -> ("dwProcImgCount"=w464:u32, "phRec out"=w468:u64, "error out"=w469:errorcluster)  [unwired: 5 in, 9 out]
                                n229 = local read "dwProcImgCount"() -> (w466:u32[])
                                n230 = Replace Array Subset(array=w466, new element=w464, index=w465) -> (w463:u32[])
                                n231 = local write "dwProcImgCount"(w463) -> ()
                                }
                              }
                            }
                            n232 = while {
                              tunnel: w451 -> [w472]
                              tunnel: [w472] -> w449
                              stop <- w473 stop-if-true
                              n233 = local read "Start recording"() -> (w473:bool)
                              n234 = Wait (ms)(milliseconds to wait=u32 100) -> ()  [unwired: 1 out]
                            }
                            n235 = property on="Init" class="Bool (strict)"("DisabledEnum"=T2."Disabled and Grayed Out" ("Disabled")) -> ()  [unwired: 2 in, 2 out]
                            n236 = property on="Start recording" class="Bool (strict)"("DisabledEnum"=T2."Enabled" ("Disabled")) -> ()  [unwired: 2 in, 2 out]
                          }
                        }
                        n237 = property on="dwImgCountArr" class="Arr (strict)"("DisabledEnum"=w434) -> ()  [unwired: 2 in, 2 out]
                        n238 = property on="wRamSegment" class="Arr (strict)"("DisabledEnum"=w434) -> ()  [unwired: 2 in, 2 out]
                        n239 = property on="wType" class="Ring (strict)"("DisabledEnum"=w434) -> ()  [unwired: 2 in, 2 out]
                        n240 = property on="baseName" class="Str"("DisabledEnum"=w434) -> ()  [unwired: 2 in, 2 out]
                        n241 = property on="Init" class="Bool (strict)"("DisabledEnum"=w434) -> ()  [unwired: 2 in, 2 out]
                        n242 = local write "Init"(FALSE ("Init")) -> ()
                        n243 = local write "Error"(w441) -> ()
                        n244 = property on="bAutoExp" class="Bool (strict)"("DisabledEnum"=w435) -> ()  [unwired: 2 in, 2 out]
                        n245 = property on="wSmoothness" class="DigNum (strict)"("DisabledEnum"=w435) -> ()  [unwired: 2 in, 2 out]
                        n246 = property on="dwMinExposure" class="DigNum (strict)"("DisabledEnum"=w435) -> ()  [unwired: 2 in, 2 out]
                        n247 = property on="dwMaxExposure" class="DigNum (strict)"("DisabledEnum"=w435) -> ()  [unwired: 2 in, 2 out]
                        n248 = property on="wExpBase" class="Ring (strict)"("DisabledEnum"=w435) -> ()  [unwired: 2 in, 2 out]
                        n249 = property on="wRegionType" class="Ring (strict)"("DisabledEnum"=w435) -> ()  [unwired: 2 in, 2 out]
                      }
                    }
                  }
                  frame #1 {
                    n250 = local read "Error"() -> (w475:errorcluster)
                    n251 = local read "Quit"() -> (w478:bool)
                    n252 = Unbundle By Name(w475) -> ("status"=w477:bool)
                    n253 = Not Or(1:w477, 2:w478) -> (0:w476:bool)
                    n254 = case shown="True" w476 {
                      tunnel: w475 -> [_ w480]
                      frame False {
                      }
                      frame True {
                        w479 = T2."Enabled" ("Disabled")
                        # "Start Record of all cameras and wait till record is finished/stopped\nGet recorder status meanwhile\nChange from 0 to valid cam handle if only one camera should be started"
                        n255 = local read "phRec"() -> (w490:u64)
                        n256 = property on="Stop recording" class="Bool (strict)"(error in=w480, "DisabledEnum"=w479) -> ()  [unwired: 1 in, 2 out]
                        n257 = property on="roiY1" class="DigNum (strict)"(error in=w480, "DisabledEnum"=w479) -> ()  [unwired: 1 in, 2 out]
                        n258 = property on="Image Height" class="DigNum (strict)"(error in=w480, "DisabledEnum"=w479) -> ()  [unwired: 1 in, 2 out]
                        n259 = property on="roiX0" class="DigNum (strict)"(error in=w480, "DisabledEnum"=w479) -> ()  [unwired: 1 in, 2 out]
                        n260 = property on="roiX1" class="DigNum (strict)"(error in=w480, "DisabledEnum"=w479) -> ()  [unwired: 1 in, 2 out]
                        n261 = property on="roiY0" class="DigNum (strict)"(error in=w480, "DisabledEnum"=w479) -> ()  [unwired: 1 in, 2 out]
                        n262 = property on="Image Width" class="DigNum (strict)"(error in=w480, "DisabledEnum"=w479) -> ()  [unwired: 1 in, 2 out]
                        n263 = property on="Cam Index" class="DigNum (strict)"(error in=w480, "DisabledEnum"=w479) -> ()  [unwired: 1 in, 2 out]
                        n264 = property on="Start recording" class="Bool (strict)"(error in=w480, "DisabledEnum"=T2."Disabled and Grayed Out" ("Disabled")) -> ()  [unwired: 1 in, 2 out]
                        n265 = call "PCO_RecorderStartRecord.vi"("error in (no error)"=w480, "phCam"=u64 0, "phRec"=w490) -> ("error out"=w483:errorcluster, "phRec out"=w481:u64)  [unwired: 6 in, 1 out]
                        n266 = local read "Quit"() -> (w485:bool)
                        n267 = Unbundle By Name(w483) -> ("status"=w486:bool)
                        n268 = Not Or(1:w486, 2:w485) -> (0:w484:bool)
                        n269 = case shown="True" w484 {
                          tunnel: w481 -> [_ w506]
                          tunnel: [w496 w501] -> w488
                          tunnel: w483 -> [w496 w505]
                          frame False {
                          }
                          frame True {
                            # "Set visible only\nto force a refresh"
                            # "Read status once again when all cameras have stopped recording"
                            # "Wait for Finish of recording"
                            n270 = property on="Image" class="IntGraph (strict)"("Frame Color"=u32 16711680, "Visible"=FALSE, "Visible"=TRUE) -> ()  [unwired: 2 in, 2 out]
                            n271 = while {
                              shift-right: [w561] -> w502
                              shift-left: w506 -> [w550]
                              shift-right: [w555] -> w504
                              shift-left: w505 -> [w548]
                              stop <- w554 stop-if-true
                              # "Get image from selected \ncamera if the camera is running"
                              # "Read status of all cameras and update values in the arrays\nBreak either when stop record is pressed or all cameras have finished"
                              n272 = local read "dwProcImgCount"() -> (w544:u32[])
                              n273 = local read "bIsRunning"() -> (w551:bool[])
                              n274 = local read "Cam Index"() -> (w543:u32)
                              n275 = local read "phCam"() -> (w546:u64[])
                              n276 = Index Array(array=w546, index=w543) -> (element=w545:u64)
                              n277 = Index Array(array=w551, index=w543) -> (element=w540:bool)
                              n278 = Index Array(array=w544, index=w543) -> (element=w542:u32)
                              n279 = Greater Than 0?(x=w542) -> (x > 0?=w541:bool)
                              n280 = And(x=w540, y=w541) -> (x .and. y?=w539:bool)
                              n281 = case shown="True" w539 {
                                tunnel: w550 -> [w563 w574]
                                tunnel: [w563 w573] -> w549
                                tunnel: w548 -> [w562 w564]
                                tunnel: [w562 w564] -> w547
                                tunnel: w545 -> [_ w572]
                                frame False {
                                }
                                frame True {
                                n282 = local read "roiX0"() -> (w571:u16)
                                n283 = local read "roiY0"() -> (w570:u16)
                                n284 = local read "roiX1"() -> (w569:u16)
                                n285 = local read "roiY1"() -> (w568:u16)
                                n286 = call "PCO_RecorderCopyImage.vi"("phRec"=w574, "phCam"=w572, "dwImgIdx"=u32 4294967295, "wRoiX0"=w571, "wRoiY0"=w570, "wRoiX1"=w569, "wRoiY1"=w568, "error in (no error)"=w564) -> ("phRec out"=w573:u64, "wImgBuf"=w566:u16[][], "error out"=w565:errorcluster)  [unwired: 13 in, 4 out]
                                n287 = local write "Image"(w566) -> ()
                                n288 = local write "Error"(w565) -> ()
                                }
                              }
                              n289 = local read "phCam"() -> (w560:u64[])
                              n290 = local read "Stop recording"() -> (w553:bool)
                              n291 = for {
                                shift-right: [w611] -> w561
                                shift-left: w549 -> [w612]
                                tunnel: w560 -> [w610] mode=indexing
                                shift-right: [w608] -> w556
                                shift-left: w547 -> [w609]
                                shift-right: [w605] -> w558
                                shift-left: FALSE ("bIsRunning out") -> [w607]
                                i -> [w582]
                                n292 = local read "bFIFOOverflow"() -> (w583:bool[])
                                n293 = local read "stopTime[ms]"() -> (w603:u32[])
                                n294 = local read "dwProcImgCount"() -> (w597:u32[])
                                n295 = local read "dwReqImgCount"() -> (w596:u32[])
                                n296 = local read "startTime[ms]"() -> (w604:u32[])
                                n297 = local read "bBuffersFull"() -> (w601:bool[])
                                n298 = local read "bIsRunning"() -> (w602:bool[])
                                n299 = local read "lastError"() -> (w595:u32[])
                                n300 = call "PCO_RecorderGetStatus.vi"("phRec"=w612, "phCam"=w610, "error in (no error)"=w609) -> ("dwStartTime"=w587:u32, "dwStopTime"=w591:u32, "bBuffersFull"=w588:bool, "bFIFOOverflow"=w581:bool, "dwProcImgCount"=w585:u32, "dwReqImgCount"=w586:u32, "phRec out"=w611:u64, "bIsRunning"=w590:bool, "dwLastError"=w589:u32, "error out"=w608:errorcluster)  [unwired: 5 in, 2 out]
                                n301 = Or(x=w590, y=w607) -> (x .or. y?=w605:bool)
                                n302 = Replace Array Subset(array=w595, new element=w589, index=w582) -> (w592:u32[])
                                n303 = Replace Array Subset(array=w604, new element=w587, index=w582) -> (w606:u32[])
                                n304 = Replace Array Subset(array=w596, new element=w586, index=w582) -> (w593:u32[])
                                n305 = Replace Array Subset(array=w603, new element=w591, index=w582) -> (w600:u32[])
                                n306 = Replace Array Subset(array=w602, new element=w590, index=w582) -> (w599:bool[])
                                n307 = Replace Array Subset(array=w601, new element=w588, index=w582) -> (w598:bool[])
                                n308 = Replace Array Subset(array=w597, new element=w585, index=w582) -> (w594:u32[])
                                n309 = Replace Array Subset(array=w583, new element=w581, index=w582) -> (w584:bool[])
                                n310 = local write "bFIFOOverflow"(w584) -> ()
                                n311 = local write "stopTime[ms]"(w600) -> ()
                                n312 = local write "dwProcImgCount"(w594) -> ()
                                n313 = local write "dwReqImgCount"(w593) -> ()
                                n314 = local write "startTime[ms]"(w606) -> ()
                                n315 = local write "bBuffersFull"(w598) -> ()
                                n316 = local write "bIsRunning"(w599) -> ()
                                n317 = local write "lastError"(w592) -> ()
                              }
                              n318 = case shown="False" w553 {
                                selector: w553 -> [w575 w578]
                                tunnel: [w575 w578] -> w552
                                tunnel: w549 -> [_ w577]
                                frame False {
                                }
                                frame True {
                                # "Stop record of all cameras"
                                n319 = call "PCO_RecorderStopRecord.vi"("phCam"=u64 0, "phRec"=w577) -> ()  [unwired: 7 in, 3 out]
                                }
                              }
                              n320 = Not(x=w558) -> (.not. x?=w557:bool)
                              n321 = Or(x=w557, y=w552) -> (x .or. y?=w554:bool)
                              n322 = flat-sequence {
                                tunnel: w556 -> [w580]
                                tunnel: [w580] -> w555
                                frame #0 {
                                n323 = Wait (ms)(milliseconds to wait=u32 100) -> ()  [unwired: 1 out]
                                }
                              }
                            }
                            n324 = local read "phCam"() -> (w503:u64[])
                            n325 = for {
                              shift-right: [w537] -> _
                              shift-left: w502 -> [w538]
                              tunnel: w503 -> [w536] mode=indexing
                              shift-right: [w534] -> w501
                              shift-left: w504 -> [w535]
                              shift-right: [w531] -> _
                              shift-left: FALSE ("bIsRunning out") -> [w533]
                              i -> [w508]
                              n326 = local read "bFIFOOverflow"() -> (w509:bool[])
                              n327 = local read "stopTime[ms]"() -> (w529:u32[])
                              n328 = local read "dwProcImgCount"() -> (w523:u32[])
                              n329 = local read "dwReqImgCount"() -> (w522:u32[])
                              n330 = local read "startTime[ms]"() -> (w530:u32[])
                              n331 = local read "bBuffersFull"() -> (w527:bool[])
                              n332 = local read "bIsRunning"() -> (w528:bool[])
                              n333 = local read "lastError"() -> (w521:u32[])
                              n334 = call "PCO_RecorderGetStatus.vi"("phRec"=w538, "phCam"=w536, "error in (no error)"=w535) -> ("dwStartTime"=w513:u32, "dwStopTime"=w517:u32, "bBuffersFull"=w514:bool, "bFIFOOverflow"=w507:bool, "dwProcImgCount"=w511:u32, "dwReqImgCount"=w512:u32, "phRec out"=w537:u64, "bIsRunning"=w516:bool, "dwLastError"=w515:u32, "error out"=w534:errorcluster)  [unwired: 5 in, 2 out]
                              n335 = Or(x=w516, y=w533) -> (x .or. y?=w531:bool)
                              n336 = Replace Array Subset(array=w521, new element=w515, index=w508) -> (w518:u32[])
                              n337 = Replace Array Subset(array=w530, new element=w513, index=w508) -> (w532:u32[])
                              n338 = Replace Array Subset(array=w522, new element=w512, index=w508) -> (w519:u32[])
                              n339 = Replace Array Subset(array=w529, new element=w517, index=w508) -> (w526:u32[])
                              n340 = Replace Array Subset(array=w528, new element=w516, index=w508) -> (w525:bool[])
                              n341 = Replace Array Subset(array=w527, new element=w514, index=w508) -> (w524:bool[])
                              n342 = Replace Array Subset(array=w523, new element=w511, index=w508) -> (w520:u32[])
                              n343 = Replace Array Subset(array=w509, new element=w507, index=w508) -> (w510:bool[])
                              n344 = local write "bFIFOOverflow"(w510) -> ()
                              n345 = local write "stopTime[ms]"(w526) -> ()
                              n346 = local write "dwProcImgCount"(w520) -> ()
                              n347 = local write "dwReqImgCount"(w519) -> ()
                              n348 = local write "startTime[ms]"(w532) -> ()
                              n349 = local write "bBuffersFull"(w524) -> ()
                              n350 = local write "bIsRunning"(w525) -> ()
                              n351 = local write "lastError"(w518) -> ()
                            }
                          }
                        }
                        n352 = local read "phRec"() -> (w489:u64)
                        n353 = flat-sequence {
                          tunnel: w482 -> [_]
                          frame #0 {
                            w492 = FALSE ("bAutoExp")
                            # "Switch off auto exposure\nSignaling to fire the event"
                            n354 = local write "Start recording"(FALSE ("Start recording")) -> ()
                            n355 = property on="Stop recording" class="Bool (strict)"("DisabledEnum"=T2."Disabled and Grayed Out" ("Disabled")) -> ()  [unwired: 2 in, 2 out]
                            n356 = property on="ResetRecorder" class="Bool (strict)"("DisabledEnum"=T2."Enabled" ("Disabled")) -> ()  [unwired: 2 in, 2 out]
                            n357 = property on="bAutoExp" class="Bool (strict)"("Value"=w492, "Val(Sgnl)"=w492) -> ()  [unwired: 2 in, 2 out]
                          }
                        }
                        n358 = case shown="Error" w488 {
                          selector: w488 -> [w613 _]
                          tunnel: w489 -> [_ w615]
                          tunnel: [w613 w614] -> w482
                          frame No Error {
                          }
                          frame Error {
                            n359 = call "PCO_RecorderDelete.vi"("phRec"=w615) -> ("error out"=w614:errorcluster)  [unwired: 9 in, 1 out]
                            n360 = flat-sequence {
                              tunnel: w614 -> [_]
                              frame #0 {
                                n361 = local write "phRec"(u64 0 ("phRec")) -> ()
                              }
                            }
                          }
                        }
                        n362 = local write "Error"(w488) -> ()
                      }
                    }
                  }
                  frame #2 {
                    n363 = local read "Error"() -> (w618:errorcluster)
                    n364 = local write "Stop recording"(FALSE ("Stop recording")) -> ()
                    n365 = local read "Quit"() -> (w620:bool)
                    n366 = Unbundle By Name(w618) -> ("status"=w619:bool)
                    n367 = Not Or(1:w619, 2:w620) -> (0:w617:bool)
                    n368 = case shown="True" w617 {
                      frame False {
                      }
                      frame True {
                        w622 = T2."Disabled and Grayed Out" ("Disabled")
                        w636 = u32 2 items=["PCO_RECORDER_MODE_FILE"=1, "PCO_RECORDER_MODE_MEMORY"=2, "PCO_RECORDER_MODE_CAMRAM"=3] ("dwRecMode")
                        w653 = T2."Enabled" ("Disabled")
                        # "Disable image index for fifo mode"
                        # "Set visible only to force a redraw"
                        # "Set visible only to force a redraw"
                        n369 = local read "Cam Index"() -> (w626:u32)
                        n370 = local read "dwRecMode"() -> (w638:u16)
                        n371 = local read "wType"() -> (w635:u16)
                        n372 = local read "dwProcImgCount"() -> (w627:u32[])
                        n373 = local read "dwReqImgCount"() -> (w646:u32[])
                        n374 = property on="bAutoExp" class="Bool (strict)"("DisabledEnum"=w622) -> ()  [unwired: 2 in, 2 out]
                        n375 = property on="wSmoothness" class="DigNum (strict)"("DisabledEnum"=w622) -> ()  [unwired: 2 in, 2 out]
                        n376 = property on="dwMinExposure" class="DigNum (strict)"("DisabledEnum"=w622) -> ()  [unwired: 2 in, 2 out]
                        n377 = property on="dwMaxExposure" class="DigNum (strict)"("DisabledEnum"=w622) -> ()  [unwired: 2 in, 2 out]
                        n378 = property on="wExpBase" class="Ring (strict)"("DisabledEnum"=w622) -> ()  [unwired: 2 in, 2 out]
                        n379 = property on="wRegionType" class="Ring (strict)"("DisabledEnum"=w622) -> ()  [unwired: 2 in, 2 out]
                        n380 = Equal?(x=u16 3, y=w635) -> (x = y?=w633:bool)
                        n381 = Equal?(x=w636, y=w638) -> (x = y?=w632:bool)
                        n382 = And(x=w632, y=w633) -> (x .and. y?=w631:bool)
                        n383 = Index Array(array=w627, index=w626) -> (element=w624:u32)
                        n384 = Index Array(array=w646, index=w626) -> (element=w625:u32)
                        n385 = case shown="True" w631 {
                          tunnel: [T2."Enabled" ("Disabled") T2."Disabled and Grayed Out" ("Disabled")] -> w637
                          frame False {
                          }
                          frame True {
                          }
                        }
                        n386 = local read "Image Height"() -> (w647:u16)
                        n387 = Max & Min(x=w625, y=w624) -> (min(x,y)=w623:u32)  [unwired: 1 out]
                        n388 = local read "Image Width"() -> (w645:u16)
                        n389 = local read "phCam"() -> (w652:u64[])
                        n390 = Array Size(array=w652) -> (size(s)=w651:i32)
                        n391 = property on="Get Image" class="Bool (strict)"("Visible"=w631) -> ()  [unwired: 2 in, 2 out]
                        n392 = property on="Image" class="IntGraph (strict)"("Frame Color"=u32 16711680, "Visible"=FALSE, "Visible"=TRUE) -> (error out=w629:errorcluster)  [unwired: 2 in, 1 out]
                        n393 = Decrement(x=w647) -> (x-1=w649:u16)
                        n394 = Decrement(x=w645) -> (x-1=w648:u16)
                        n395 = Decrement(x=w651) -> (x-1=w650:i32)
                        n396 = Decrement(x=w623) -> (x-1=w644:u32)
                        n397 = property on="roiX0" class="DigNum (strict)"("DisabledEnum"=w653, "Maximum"=w648) -> ()  [unwired: 2 in, 2 out]
                        n398 = property on="roiX1" class="DigNum (strict)"("DisabledEnum"=w653, "Maximum"=w645) -> ()  [unwired: 2 in, 2 out]
                        n399 = property on="roiY0" class="DigNum (strict)"("DisabledEnum"=w653, "Maximum"=w649) -> ()  [unwired: 2 in, 2 out]
                        n400 = property on="roiY1" class="DigNum (strict)"("DisabledEnum"=w653, "Maximum"=w647) -> ()  [unwired: 2 in, 2 out]
                        n401 = property on="Cam Index" class="DigNum (strict)"("DisabledEnum"=w653, "Maximum"=w650) -> ()  [unwired: 2 in, 2 out]
                        n402 = property on="Image Index" class="DigNum (strict)"("DisabledEnum"=w637, "Maximum"=w644) -> ()  [unwired: 2 in, 2 out]
                        n403 = while {
                          tunnel: w631 -> [w658]
                          tunnel: w629 -> [w656]
                          tunnel: [w656] -> w628
                          stop <- w660 stop-if-true
                          n404 = flat-sequence {
                            tunnel: w658 -> [w664]
                            tunnel: [w664] -> w657
                            tunnel: [w670] -> w663
                            tunnel: w657 -> [w669]
                            frame #0 {
                              n405 = Wait (ms)(milliseconds to wait=u32 100) -> ()  [unwired: 1 out]
                            }
                            frame #1 {
                              # "Read images until stop button is pressed\nGet image size of current camera and adapt roi accordingly\nCopy image inside roi into image buffer and show it on display"
                              n406 = local read "Cam Index"() -> (w671:u32)
                              n407 = local read "phCam"() -> (w672:u64[])
                              n408 = local read "phRec"() -> (w667:u64)
                              n409 = local read "Error"() -> (w666:errorcluster)
                              n410 = Index Array(array=w672, index=w671) -> (element=w668:u64)
                              n411 = flat-sequence {
                                tunnel: [w677] -> w670
                                tunnel: w669 -> [w676]
                                tunnel: w668 -> [w675]
                                tunnel: w667 -> [w674]
                                tunnel: w666 -> [w673]
                                frame #0 {
                                # "FIFO Mode ?"
                                # "If FIFO Mode, use button to get next image, not auto readout"
                                n412 = case shown="True" w676 {
                                tunnel: [w678 w688] -> w677
                                tunnel: w674 -> [w681 w692]
                                tunnel: w675 -> [w680 w691]
                                tunnel: w673 -> [w679 w690]
                                frame False {
                                n413 = local read "Image Index"() -> (w686:u32)
                                n414 = local read "roiX0"() -> (w685:u16)
                                n415 = local read "roiY0"() -> (w684:u16)
                                n416 = local read "roiX1"() -> (w683:u16)
                                n417 = local read "roiY1"() -> (w682:u16)
                                n418 = call "PCO_RecorderCopyImage.vi"("phRec"=w681, "phCam"=w680, "dwImgIdx"=w686, "wRoiX0"=w685, "wRoiY0"=w684, "wRoiX1"=w683, "wRoiY1"=w682, "error in (no error)"=w679) -> ("wImgBuf"=w687:u16[][], "error out"=w678:errorcluster)  [unwired: 13 in, 5 out]
                                n419 = local write "Image"(w687) -> ()
                                n420 = local write "Error"(w678) -> ()
                                }
                                frame True {
                                # "In FIFO mode image is only read when button is pressed"
                                n421 = local read "Get Image"() -> (w689:bool)
                                n422 = case shown="True" w689 {
                                tunnel: w692 -> [_ w706]
                                tunnel: w691 -> [_ w701]
                                tunnel: w690 -> [w693 w700]
                                tunnel: [w693 w697] -> w688
                                frame False {
                                }
                                frame True {
                                # "If no more images available\njust quit loop with Mbx"
                                # "Reset Button"
                                # "Always use index 0\nfor FIFO mode"
                                n423 = local write "Get Image"(FALSE ("Get Image")) -> ()
                                n424 = local read "roiX0"() -> (w705:u16)
                                n425 = local read "roiY0"() -> (w704:u16)
                                n426 = local read "roiX1"() -> (w703:u16)
                                n427 = local read "roiY1"() -> (w702:u16)
                                n428 = call "PCO_RecorderCopyImage.vi"("phRec"=w706, "phCam"=w701, "dwImgIdx"=u32 0 ("Image Index"), "wRoiX0"=w705, "wRoiY0"=w704, "wRoiX1"=w703, "wRoiY1"=w702, "error in (no error)"=w700) -> ("ErrorMessage"=w695:i32, "wImgBuf"=w707:u16[][], "error out"=w697:errorcluster)  [unwired: 13 in, 4 out]
                                n429 = local write "Image"(w707) -> ()
                                n430 = Equal?(x=w695, y=-2147471324 ("ErrorMessage")) -> (x = y?=w694:bool)
                                n431 = case shown="True" w694 {
                                tunnel: w697 -> [w708 _]
                                frame False {
                                n432 = local write "Error"(w708) -> ()
                                }
                                frame True {
                                n433 = One Button Dialog(message="No more images\navailable") -> ()  [unwired: 1 in, 1 out]
                                }
                                }
                                }
                                }
                                }
                                }
                                }
                              }
                            }
                          }
                          n434 = local read "ResetRecorder"() -> (w661:bool)
                          n435 = Unbundle By Name(w663) -> ("status"=w662:bool)
                          n436 = local read "Quit"() -> (w659:bool)
                          n437 = Compound Arithmetic op=OR(w662, w661, w659) -> (w660:bool)
                        }
                        n438 = property on="Image" class="IntGraph (strict)"(error in=w628, "Frame Color"=u32 14869218, "Visible"=FALSE, "Visible"=TRUE) -> ()  [unwired: 1 in, 2 out]
                      }
                    }
                  }
                  frame #3 {
                    w711 = T2."Disabled and Grayed Out" ("Disabled")
                    w712 = T2."Disabled and Grayed Out" ("Disabled")
                    n439 = local read "Error"() -> (w713:errorcluster)
                    n440 = local read "Quit"() -> (w716:bool)
                    n441 = Unbundle By Name(w713) -> ("status"=w715:bool)
                    n442 = property on="Cam Index" class="DigNum (strict)"("DisabledEnum"=w712) -> ()  [unwired: 2 in, 2 out]
                    n443 = property on="Image Index" class="DigNum (strict)"("DisabledEnum"=w712) -> ()  [unwired: 2 in, 2 out]
                    n444 = property on="roiX0" class="DigNum (strict)"("DisabledEnum"=w712) -> ()  [unwired: 2 in, 2 out]
                    n445 = property on="roiX1" class="DigNum (strict)"("DisabledEnum"=w712) -> ()  [unwired: 2 in, 2 out]
                    n446 = property on="roiY0" class="DigNum (strict)"("DisabledEnum"=w712) -> ()  [unwired: 2 in, 2 out]
                    n447 = property on="roiY1" class="DigNum (strict)"("DisabledEnum"=w712) -> ()  [unwired: 2 in, 2 out]
                    n448 = property on="Image Height" class="DigNum (strict)"("DisabledEnum"=w712) -> ()  [unwired: 2 in, 2 out]
                    n449 = property on="Image Width" class="DigNum (strict)"("DisabledEnum"=w712) -> ()  [unwired: 2 in, 2 out]
                    n450 = local write "ResetRecorder"(FALSE ("Quit")) -> ()
                    n451 = Not Or(1:w715, 2:w716) -> (0:w714:bool)
                    n452 = property on="bAutoExp" class="Bool (strict)"("DisabledEnum"=w711, "Value"=FALSE ("bAutoExp")) -> ()  [unwired: 2 in, 2 out]
                    n453 = property on="wSmoothness" class="DigNum (strict)"("DisabledEnum"=w711) -> ()  [unwired: 2 in, 2 out]
                    n454 = property on="dwMinExposure" class="DigNum (strict)"("DisabledEnum"=w711) -> ()  [unwired: 2 in, 2 out]
                    n455 = property on="dwMaxExposure" class="DigNum (strict)"("DisabledEnum"=w711) -> ()  [unwired: 2 in, 2 out]
                    n456 = property on="wExpBase" class="Ring (strict)"("DisabledEnum"=w711) -> ()  [unwired: 2 in, 2 out]
                    n457 = property on="wRegionType" class="Ring (strict)"("DisabledEnum"=w711) -> ()  [unwired: 2 in, 2 out]
                    n458 = case shown="True" w714 {
                      tunnel: w713 -> [_ w719]
                      frame False {
                      }
                      frame True {
                        # "Delete Recorder"
                        n459 = local read "phRec"() -> (w718:u64)
                        n460 = call "PCO_RecorderDelete.vi"("error in (no error)"=w719, "phRec"=w718) -> ("error out"=w720:errorcluster)  [unwired: 8 in, 1 out]
                        n461 = call "Simple Error Handler.vi"("error in (no error)"=w720) -> ()  [unwired: 4 in, 5 out]
                        n462 = local write "Error"(w720) -> ()
                        n463 = flat-sequence {
                          tunnel: w720 -> [_]
                          frame #0 {
                            n464 = local write "phRec"(u64 0 ("phRec")) -> ()
                          }
                        }
                        n465 = property on="ResetRecorder" class="Bool (strict)"("DisabledEnum"=T2."Disabled and Grayed Out" ("Disabled")) -> ()  [unwired: 2 in, 2 out]
                      }
                    }
                  }
                }
              }
            }
          }
        }
      }
      n466 = while {
        stop <- w11 stop-if-true
        # "Event structure for parameter checking"
        n467 = event shown="[1] \"dwMinExposure\": Value Change" {
          selector: _ -> [_ _ _ _ _ _ _ _ _ _ _ _ _ _]
          dyn-events: _ -> [_ _ _ _ _ _ _ _ _ _ _ _ _ _]
          timeout: 1000 -> [_ _ _ _ _ _ _ _ _ _ _ _ _ _]
          tunnel: [_ _ _ _ _ _ TRUE _ _ _ _ _ _ _] -> w11
          event Timeout {
            n468 = event-data() -> ()  [unwired: 1 in, 3 out]
          }
          event "dwMinExposure": Value Change {
            n469 = event-data() -> ()  [unwired: 1 in, 6 out]
            n470 = local read "phRec"() -> (w13:u64)
            n471 = Greater Than 0?(x=w13) -> (x > 0?=w14:bool)
            n472 = case shown="True" w14 {
              tunnel: w13 -> [_ w16]
              frame False {
              }
              frame True {
                n473 = flat-sequence {
                  tunnel: w16 -> [w23]
                  tunnel: [w23] -> w15
                  tunnel: [w28] -> w17
                  tunnel: w15 -> [w28]
                  tunnel: w17 -> [w33]
                  frame #0 {
                    n474 = local read "exposureMaxLimit"() -> (w18:u64)
                    n475 = local read "exposureMinLimit"() -> (w19:u64)
                    n476 = local read "dwMinExposure"() -> (w20:u32)
                    n477 = Less?(x=w20, y=w19) -> (x < y?=w22:bool)
                    n478 = Greater Or Equal?(x=w20, y=w18) -> (x >= y?=w21:bool)
                    n479 = case shown="True" w22 {
                      tunnel: w19 -> [_ w26]
                      frame False {
                      }
                      frame True {
                        n480 = local write "dwMinExposure"(w26) -> ()
                      }
                    }
                    n481 = case shown="True" w21 {
                      tunnel: w18 -> [_ w25]
                      frame False {
                      }
                      frame True {
                        n482 = Decrement(x=w25) -> (x-1=w24:u64)
                        n483 = local write "dwMinExposure"(w24) -> ()
                      }
                    }
                  }
                  frame #1 {
                    n484 = local read "dwMaxExposure"() -> (w29:u32)
                    n485 = local read "dwMinExposure"() -> (w27:u32)
                    n486 = Greater Or Equal?(x=w27, y=w29) -> (x >= y?=w30:bool)
                    n487 = case shown="True" w30 {
                      tunnel: w27 -> [_ w31]
                      frame False {
                      }
                      frame True {
                        n488 = Increment(x=w31) -> (x+1=w32:u32)
                        n489 = local write "dwMaxExposure"(w32) -> ()
                      }
                    }
                  }
                  frame #2 {
                    n490 = local read "phCam"() -> (w34:u64[])
                    n491 = for {
                      tunnel: w33 -> [w35]
                      tunnel: [w36] -> _ mode=indexing
                      tunnel: w34 -> [w36] mode=indexing
                      # "Here we set the same settings for all cameras\nbut you could also use different settings for different cameras\nOr just activate/deactivate it for specific cameras"
                      n492 = local read "dwMinExposure"() -> (w38:u32)
                      n493 = local read "wSmoothness"() -> (w41:u16)
                      n494 = local read "wExpBase"() -> (w39:u16)
                      n495 = local read "bAutoExp"() -> (w42:bool)
                      n496 = local read "Error"() -> (w37:errorcluster)
                      n497 = local read "dwMaxExposure"() -> (w40:u32)
                      n498 = call "PCO_RecorderSetAutoExposure.vi"("phRec"=w35, "dwMinExposure"=w38, "wExpBase"=w39, "phCam"=w36, "bAutoExpState"=w42, "wSmoothness"=w41, "error in (no error)"=w37, "dwMaxExposure"=w40) -> ("error out"=w43:errorcluster)  [unwired: 5 in, 2 out]
                      n499 = local write "Error"(w43) -> ()
                    }
                  }
                }
              }
            }
          }
          event "dwMaxExposure": Value Change {
            n500 = event-data() -> ()  [unwired: 1 in, 6 out]
            n501 = local read "phRec"() -> (w44:u64)
            n502 = Greater Than 0?(x=w44) -> (x > 0?=w45:bool)
            n503 = case shown="True" w45 {
              tunnel: w44 -> [_ w47]
              frame False {
              }
              frame True {
                n504 = flat-sequence {
                  tunnel: w47 -> [w54]
                  tunnel: [w54] -> w46
                  tunnel: [w58] -> w48
                  tunnel: w46 -> [w58]
                  tunnel: w48 -> [w64]
                  frame #0 {
                    n505 = local read "exposureMaxLimit"() -> (w49:u64)
                    n506 = local read "exposureMinLimit"() -> (w50:u64)
                    n507 = local read "dwMaxExposure"() -> (w51:u32)
                    n508 = Less Or Equal?(x=w51, y=w50) -> (x <= y?=w52:bool)
                    n509 = Greater?(x=w51, y=w49) -> (0:w53:bool)
                    n510 = case shown="True" w52 {
                      tunnel: w50 -> [_ w57]
                      frame False {
                      }
                      frame True {
                        n511 = Increment(x=w57) -> (x+1=w56:u64)
                        n512 = local write "dwMaxExposure"(w56) -> ()
                      }
                    }
                    n513 = case shown="True" w53 {
                      tunnel: w49 -> [_ w55]
                      frame False {
                      }
                      frame True {
                        n514 = local write "dwMaxExposure"(w55) -> ()
                      }
                    }
                  }
                  frame #1 {
                    n515 = local read "dwMaxExposure"() -> (w59:u32)
                    n516 = local read "dwMinExposure"() -> (w61:u32)
                    n517 = Greater Or Equal?(x=w61, y=w59) -> (x >= y?=w60:bool)
                    n518 = case shown="True" w60 {
                      tunnel: w59 -> [_ w62]
                      frame False {
                      }
                      frame True {
                        n519 = Decrement(x=w62) -> (x-1=w63:u32)
                        n520 = local write "dwMinExposure"(w63) -> ()
                      }
                    }
                  }
                  frame #2 {
                    n521 = local read "phCam"() -> (w65:u64[])
                    n522 = for {
                      tunnel: w64 -> [w66]
                      tunnel: [w67] -> _ mode=indexing
                      tunnel: w65 -> [w67] mode=indexing
                      # "Here we set the same settings for all cameras\nbut you could also use different settings for different cameras\nOr just activate/deactivate it for specific cameras"
                      n523 = local read "dwMinExposure"() -> (w69:u32)
                      n524 = local read "wSmoothness"() -> (w72:u16)
                      n525 = local read "wExpBase"() -> (w70:u16)
                      n526 = local read "bAutoExp"() -> (w73:bool)
                      n527 = local read "Error"() -> (w68:errorcluster)
                      n528 = local read "dwMaxExposure"() -> (w71:u32)
                      n529 = call "PCO_RecorderSetAutoExposure.vi"("phRec"=w66, "dwMinExposure"=w69, "wExpBase"=w70, "phCam"=w67, "bAutoExpState"=w73, "wSmoothness"=w72, "error in (no error)"=w68, "dwMaxExposure"=w71) -> ("error out"=w74:errorcluster)  [unwired: 5 in, 2 out]
                      n530 = local write "Error"(w74) -> ()
                    }
                  }
                }
              }
            }
          }
          event "bAutoExp", "wSmoothness": Value Change {
            n531 = event-data() -> ()  [unwired: 1 in, 6 out]
            n532 = local read "phRec"() -> (w75:u64)
            n533 = Greater Than 0?(x=w75) -> (x > 0?=w76:bool)
            n534 = case shown="True" w76 {
              tunnel: w75 -> [_ w77]
              frame False {
              }
              frame True {
                n535 = local read "phCam"() -> (w78:u64[])
                n536 = for {
                  tunnel: w77 -> [w79]
                  tunnel: [w80] -> _ mode=indexing
                  tunnel: w78 -> [w80] mode=indexing
                  # "Here we set the same settings for all cameras\nbut you could also use different settings for different cameras\nOr just activate/deactivate it for specific cameras"
                  n537 = local read "dwMinExposure"() -> (w82:u32)
                  n538 = local read "wSmoothness"() -> (w85:u16)
                  n539 = local read "wExpBase"() -> (w83:u16)
                  n540 = local read "bAutoExp"() -> (w86:bool)
                  n541 = local read "Error"() -> (w81:errorcluster)
                  n542 = local read "dwMaxExposure"() -> (w84:u32)
                  n543 = call "PCO_RecorderSetAutoExposure.vi"("phRec"=w79, "dwMinExposure"=w82, "wExpBase"=w83, "phCam"=w80, "bAutoExpState"=w86, "wSmoothness"=w85, "error in (no error)"=w81, "dwMaxExposure"=w84) -> ("error out"=w87:errorcluster)  [unwired: 5 in, 2 out]
                  n544 = local write "Error"(w87) -> ()
                }
              }
            }
          }
          event "wExpBase": Value Change {
            w112 = u16 1000 ("x")
            # "Force changed event"
            # "Min Exp is in ns\nMaxExp is in ms"
            n545 = event-data() -> ("OldVal"=w115:u16, "NewVal"=w92:u16)  [unwired: 1 in, 4 out]
            n546 = Subtract(x=0.0, y=w92) -> (x-y=w114:i32)
            n547 = Subtract(x=2.0, y=w92) -> (x-y=w113:i32)
            n548 = Power Of X(1:w112, 2:w114) -> (0:w108:dbl)
            n549 = Power Of X(1:w112, 2:w113) -> (0:w109:dbl)
            n550 = local read "strSensor"() -> (w111:T1)
            n551 = Unbundle By Name(w111) -> ("PCO_Description"=w110:T4)
            n552 = Unbundle By Name(w110) -> ("dwMinExposureDESC"=w107:u32, "dwMaxExposureDESC"=w106:u32)
            n553 = Subtract(x=w115, y=w92) -> (x-y=w102:i32)
            n554 = Multiply(x=w107, y=w108) -> (x*y=w91:dbl)
            n555 = Multiply(x=w106, y=w109) -> (x*y=w89:dbl)
            n556 = local read "dwMinExposure"() -> (w103:u32)
            n557 = local read "dwMaxExposure"() -> (w104:u32)
            n558 = Round Toward -Infinity(1:w89) -> (0:w88:dbl)
            n559 = Round Toward +Infinity(x=w91) -> (ceil(x): smallest int >= x=w90:dbl)
            n560 = Power Of X(1:u16 1000 ("x"), 2:w102) -> (0:w105:dbl)
            n561 = Multiply(x=w105, y=w104) -> (x*y=w97:dbl)
            n562 = Multiply(x=w103, y=w105) -> (x*y=w100:dbl)
            n563 = local write "exposureMinLimit"(w90) -> ()
            n564 = local write "exposureMaxLimit"(w88) -> ()
            n565 = Greater?(x=w97, y=w88) -> (0:w98:bool)
            n566 = Less?(x=w100, y=w90) -> (x < y?=w99:bool)
            n567 = case shown="True" w99 {
              tunnel: w90 -> [_ w119]
              tunnel: w100 -> [w118 _]
              tunnel: [w118 w119] -> w96
              frame False {
              }
              frame True {
              }
            }
            n568 = case shown="False" w98 {
              tunnel: w97 -> [w116 _]
              tunnel: w88 -> [_ w117]
              tunnel: [w116 w117] -> w95
              frame False {
              }
              frame True {
              }
            }
            n569 = local write "dwMinExposure"(w96) -> ()
            n570 = local write "dwMaxExposure"(w95) -> ()
            n571 = property on="dwMaxExposure" class="DigNum (strict)"("Val(Sgnl)"=w95) -> ()  [unwired: 2 in, 2 out]
            n572 = property on="dwMinExposure" class="DigNum (strict)"("Val(Sgnl)"=w96) -> ()  [unwired: 2 in, 2 out]
          }
          event "wRegionType": Value Change {
            n573 = event-data() -> ("NewVal"=w120:u16)  [unwired: 1 in, 5 out]
            n574 = local read "phRec"() -> (w121:u64)
            n575 = Greater Than 0?(x=w121) -> (x > 0?=w122:bool)
            n576 = case shown="True" w122 {
              tunnel: w121 -> [_ w125]
              tunnel: w120 -> [_ w123]
              frame False {
              }
              frame True {
                n577 = local read "phCam"() -> (w124:u64[])
                n578 = for {
                  tunnel: w125 -> [w137]
                  tunnel: [w127] -> _ mode=indexing
                  tunnel: w124 -> [w127] mode=indexing
                  tunnel: w123 -> [w126]
                  # "Default array since we do not use \ncustom region here"
                  # "Here we set the same settings for all cameras, but you could also use different settings for different cameras\nOr just activate/deactivate it for specific cameras"
                  n579 = local read "Error"() -> (w136:errorcluster)
                  n580 = Initialize Array(u16 0 ("element"), 1 ("dimension size")) -> (w128:u16[])
                  n581 = call "PCO_RecorderSetAutoExpRegions.vi"("phRec"=w137, "wRoiY0Arr"=w128, "phCam"=w127, "wRegionType"=w126, "wRoiX0Arr"=w128, "error in (no error)"=w136) -> ("phRec out"=w132:u64, "ErrorMessage"=w133:i32, "error out"=w130:errorcluster)  [unwired: 7 in]
                  n582 = Not Equal To 0?(x=w133) -> (x != 0?=w131:bool)
                  n583 = case shown="False" w131 {
                    tunnel: w132 -> [_ w143]
                    tunnel: w130 -> [w138 _]
                    tunnel: [w138 w141] -> w129
                    tunnel: w128 -> [_ w140]
                    tunnel: w127 -> [_ w139]
                    frame False {
                    }
                    frame True {
                      w142 = u16 3 items=["REGION_TYPE_BALANCED", "REGION_TYPE_CENTER_BASED", "REGION_TYPE_CORNER_BASED", "REGION_TYPE_FULL", "REGION_TYPE_CUSTOM"] ("wRegionType")
                      # "Set full as default region\nif an error ocurred"
                      n584 = call "PCO_RecorderSetAutoExpRegions.vi"("phRec"=w143, "wRoiY0Arr"=w140, "phCam"=w139, "wRegionType"=w142, "wRoiX0Arr"=w140) -> ("error out"=w141:errorcluster)  [unwired: 8 in, 2 out]
                      n585 = local write "wRegionType"(w142) -> ()
                    }
                  }
                  n586 = local write "Error"(w129) -> ()
                }
              }
            }
          }
          event "Quit": Value Change {
            n587 = event-data() -> ()  [unwired: 1 in, 6 out]
          }
          event "Cam Index": Value Change {
            n588 = event-data() -> ("NewVal"=w148:u32)  [unwired: 1 in, 5 out]
            n589 = local read "phCam"() -> (w165:u64[])
            n590 = local read "phRec"() -> (w166:u64)
            n591 = local read "dwProcImgCount"() -> (w149:u32[])
            n592 = local read "dwReqImgCount"() -> (w168:u32[])
            n593 = Index Array(array=w165, index=w148) -> (element=w164:u64)
            n594 = call "PCO_RecorderGetSettings.vi"("phRec"=w166, "phCam"=w164) -> ("wHeight"=w158:u16, "wWidth"=w159:u16)  [unwired: 5 in, 7 out]
            n595 = Index Array(array=w149, index=w148) -> (element=w145:u32)
            n596 = Index Array(array=w168, index=w148) -> (element=w146:u32)
            n597 = Max & Min(x=w146, y=w145) -> (min(x,y)=w147:u32)  [unwired: 1 out]
            n598 = local write "Image Height"(w158) -> ()
            n599 = local write "Image Width"(w159) -> ()
            n600 = Decrement(x=w147) -> (x-1=w167:u32)
            n601 = property on="Image Index" class="DigNum (strict)"("Maximum"=w167) -> ()  [unwired: 2 in, 2 out]
            n602 = Decrement(x=w158) -> (x-1=w163:u16)
            n603 = Decrement(x=w159) -> (x-1=w162:u16)
            n604 = property on="roiY1" class="DigNum (strict)"("Maximum"=w158) -> ()  [unwired: 2 in, 2 out]
            n605 = property on="roiY0" class="DigNum (strict)"("Maximum"=w163) -> ()  [unwired: 2 in, 2 out]
            n606 = property on="roiX0" class="DigNum (strict)"("Maximum"=w162) -> ()  [unwired: 2 in, 2 out]
            n607 = property on="roiX1" class="DigNum (strict)"("Maximum"=w159) -> ()  [unwired: 2 in, 2 out]
            n608 = local read "roiY1"() -> (w153:u16)
            n609 = local read "roiX1"() -> (w152:u16)
            n610 = Greater?(x=w153, y=w158) -> (0:w161:bool)
            n611 = Greater?(x=w152, y=w159) -> (0:w160:bool)
            n612 = case shown="False" w161 {
              tunnel: w158 -> [_ w176]
              tunnel: w153 -> [w175 _]
              tunnel: [w175 w176] -> w150
              frame False {
              }
              frame True {
                n613 = local write "roiY1"(w176) -> ()
              }
            }
            n614 = case shown="False" w160 {
              tunnel: w159 -> [_ w174]
              tunnel: w152 -> [w173 _]
              tunnel: [w173 w174] -> w151
              frame False {
              }
              frame True {
                n615 = local write "roiX1"(w174) -> ()
              }
            }
            n616 = local read "roiY0"() -> (w155:u16)
            n617 = local read "roiX0"() -> (w156:u16)
            n618 = Greater Or Equal?(x=w155, y=w150) -> (x >= y?=w154:bool)
            n619 = Greater Or Equal?(x=w156, y=w151) -> (x >= y?=w157:bool)
            n620 = case shown="True" w154 {
              tunnel: w150 -> [_ w172]
              frame False {
              }
              frame True {
                n621 = Decrement(x=w172) -> (x-1=w171:u16)
                n622 = local write "roiY0"(w171) -> ()
              }
            }
            n623 = case shown="True" w157 {
              tunnel: w151 -> [_ w170]
              frame False {
              }
              frame True {
                n624 = Decrement(x=w170) -> (x-1=w169:u16)
                n625 = local write "roiX0"(w169) -> ()
              }
            }
          }
          event "Image Width": Value Change {
            n626 = event-data() -> ("NewVal"=w177:u16)  [unwired: 1 in, 5 out]
            n627 = Decrement(x=w177) -> (x-1=w178:u16)
            n628 = property on="roiX0" class="DigNum (strict)"("Maximum"=w178) -> ()  [unwired: 2 in, 2 out]
            n629 = property on="roiX1" class="DigNum (strict)"("Maximum"=w177) -> ()  [unwired: 2 in, 2 out]
          }
          event "Image Height": Value Change {
            n630 = event-data() -> ("NewVal"=w179:u16)  [unwired: 1 in, 5 out]
            n631 = Decrement(x=w179) -> (x-1=w180:u16)
            n632 = property on="roiY1" class="DigNum (strict)"("Maximum"=w179) -> ()  [unwired: 2 in, 2 out]
            n633 = property on="roiY0" class="DigNum (strict)"("Maximum"=w180) -> ()  [unwired: 2 in, 2 out]
          }
          event "roiX0": Value Change {
            n634 = event-data() -> ("NewVal"=w181:u16)  [unwired: 1 in, 5 out]
            n635 = local read "roiX1"() -> (w183:u16)
            n636 = Greater Or Equal?(x=w181, y=w183) -> (x >= y?=w182:bool)
            n637 = case shown="False" w182 {
              tunnel: w181 -> [_ w185]
              frame False {
              }
              frame True {
                n638 = Increment(x=w185) -> (x+1=w184:u16)
                n639 = local write "roiX1"(w184) -> ()
              }
            }
          }
          event "roiY0": Value Change {
            n640 = event-data() -> ("NewVal"=w186:u16)  [unwired: 1 in, 5 out]
            n641 = local read "roiY1"() -> (w188:u16)
            n642 = Greater Or Equal?(x=w186, y=w188) -> (x >= y?=w187:bool)
            n643 = case shown="True" w187 {
              tunnel: w186 -> [_ w190]
              frame False {
              }
              frame True {
                n644 = Increment(x=w190) -> (x+1=w189:u16)
                n645 = local write "roiY1"(w189) -> ()
              }
            }
          }
          event "roiX1": Value Change {
            n646 = event-data() -> ("NewVal"=w191:u16)  [unwired: 1 in, 5 out]
            n647 = local read "roiX0"() -> (w193:u16)
            n648 = Less Or Equal?(x=w191, y=w193) -> (x <= y?=w192:bool)
            n649 = case shown="True" w192 {
              tunnel: w191 -> [_ w195]
              frame False {
              }
              frame True {
                n650 = Decrement(x=w195) -> (x-1=w194:u16)
                n651 = local write "roiX0"(w194) -> ()
              }
            }
          }
          event "roiY1": Value Change {
            n652 = event-data() -> ("NewVal"=w196:u16)  [unwired: 1 in, 5 out]
            n653 = local read "roiY0"() -> (w198:u16)
            n654 = Less Or Equal?(x=w196, y=w198) -> (x <= y?=w197:bool)
            n655 = case shown="True" w197 {
              tunnel: w196 -> [_ w200]
              frame False {
              }
              frame True {
                n656 = Decrement(x=w200) -> (x-1=w199:u16)
                n657 = local write "roiY0"(w199) -> ()
              }
            }
          }
        }
      }
    }
    frame Error {
      n658 = local write "Quit"(TRUE ("Quit")) -> ()
    }
  }
  n659 = while {
    tunnel: [w724] -> w4
    stop <- w724 stop-if-true
    n660 = event shown="[0] Panel Close?" {
      selector: _ -> [w728 w734 w737 w741]
      dyn-events: [w728 w734 w737 w741] -> _
      timeout: 1000 -> [_ _ _ _]
      tunnel: [_ w732 _ _] -> w724
      event Panel Close? {
        n661 = event-data() -> ()  [unwired: 1 in, 1 out]
        n662 = One Button Dialog(message="Please click on \"Quit Application\"\nbutton before closing!") -> (true=w726:bool)  [unwired: 1 in]
        n663 = event-data("Discard?"=w726) -> ()  [unwired: 1 in, 1 out]
      }
      event Timeout {
        # "Stop reading images if necessary"
        n664 = event-data() -> ()  [unwired: 1 in, 3 out]
        n665 = local read "Quit"() -> (w732:bool)
        n666 = property on="ResetRecorder" class="Bool (strict)"() -> ("DisabledEnum"=w730:T2)  [unwired: 2 in, 2 out]
        n667 = Equal?(x=w730, y=T2."Enabled" ("Disabled")) -> (x = y?=w729:bool)
        n668 = And(x=w729, y=w732) -> (x .and. y?=w733:bool)
        n669 = case shown="False" w733 {
          frame False {
          }
          frame True {
            n670 = flat-sequence {
              frame #0 {
                n671 = local write "ResetRecorder"(TRUE ("Stop Copy")) -> ()
              }
              frame #1 {
                n672 = Wait (ms)(milliseconds to wait=u32 1000) -> ()  [unwired: 1 out]
              }
            }
          }
        }
      }
      event "dwRecMode": Value Change {
        w740 = u32 1 items=["PCO_RECORDER_MODE_FILE"=1, "PCO_RECORDER_MODE_MEMORY_SEQUENCE"=2, "PCO_RECORDER_MODE_MEMORY_RINGBUF"=4] ("dwRecMode")
        n673 = event-data() -> ("NewVal"=w739:u16)  [unwired: 1 in, 5 out]
        n674 = Equal?(x=w740, y=w739) -> (x = y?=w738:bool)
        n675 = property on="szPath" class="Path"("Visible"=w738) -> ()  [unwired: 2 in, 2 out]
        n676 = property on="baseName" class="Str"("Visible"=w738) -> ()  [unwired: 2 in, 2 out]
      }
      event "Quit": Value Change {
        n677 = event-data() -> ("NewVal"=w742:bool)  [unwired: 1 in, 5 out]
        n678 = case shown="True" w742 {
          frame False {
          }
          frame True {
            n679 = local read "Start recording"() -> (w743:bool)
            n680 = case shown="False" w743 {
              frame False {
              }
              frame True {
                n681 = One Button Dialog(message="Please stop acquisition before closing") -> ()  [unwired: 1 in, 1 out]
                n682 = local write "Quit"(FALSE ("Quit")) -> ()
              }
            }
          }
        }
      }
    }
  }
  n683 = case shown="True" w4 {
    selector: w4 -> [w746 w748]
    tunnel: [w746 w748] -> w1
    frame False {
    }
    frame True {
      w747 = T2."Disabled and Grayed Out" ("Disabled")
      # "Reset Quit button"
      n684 = local read "phRec"() -> (w750:u64)
      n685 = local write "Quit"(FALSE ("Quit")) -> ()
      n686 = property on="ResetRecorder" class="Bool (strict)"("DisabledEnum"=w747) -> ()  [unwired: 2 in, 2 out]
      n687 = property on="dwImgDistributionArr" class="Arr (strict)"("DisabledEnum"=w747) -> ()  [unwired: 2 in, 2 out]
      n688 = property on="Create" class="Bool (strict)"("DisabledEnum"=w747) -> ()  [unwired: 2 in, 2 out]
      n689 = property on="szPath" class="Path"("DisabledEnum"=w747) -> ()  [unwired: 2 in, 2 out]
      n690 = property on="dwRecMode" class="Ring (strict)"("DisabledEnum"=w747) -> ()  [unwired: 2 in, 2 out]
      n691 = property on="dwMaxImgCountArr" class="Arr (strict)"("DisabledEnum"=w747) -> ()  [unwired: 2 in, 2 out]
      n692 = flat-sequence {
        tunnel: w750 -> [w753]
        tunnel: [w764] -> w749
        tunnel: w749 -> [w770]
        frame #0 {
          n693 = Not Equal To 0?(x=w753) -> (x != 0?=w752:bool)
          n694 = case shown="True" w752 {
            frame False {
            }
            frame True {
              n695 = flat-sequence {
                frame #0 {
                  # "Wait for finish acquisition"
                  n696 = while {
                    stop <- w754 continue-if-true
                    n697 = local read "bIsRunning"() -> (w756:bool[])
                    n698 = for {
                      tunnel: w756 -> [w759] mode=indexing
                      shift-right: [w757] -> w754
                      shift-left: FALSE -> [w758]
                      n699 = Or(x=w759, y=w758) -> (x .or. y?=w757:bool)
                    }
                  }
                }
                frame #1 {
                  n700 = local read "phRec"() -> (w762:u64)
                  n701 = local read "Error"() -> (w760:errorcluster)
                  n702 = call "PCO_RecorderDelete.vi"("phRec"=w762) -> ("error out"=w761:errorcluster)  [unwired: 9 in, 1 out]
                  n703 = case shown="No Error" w760 {
                    tunnel: w761 -> [w763 _]
                    frame No Error {
                      n704 = local write "Error"(w763) -> ()
                    }
                    frame Error {
                    }
                  }
                }
              }
            }
          }
        }
        frame #1 {
          # "Close all opened cameras in the end"
          n705 = local write "phRec"(u64 0 ("phRec")) -> ()
          n706 = local read "phCam"() -> (w764:u64[])
          n707 = for {
            tunnel: w764 -> [w766] mode=indexing
            n708 = Not Equal To 0?(x=w766) -> (x != 0?=w767:bool)
            n709 = case shown="True" w767 {
              tunnel: w766 -> [_ w768]
              frame False {
              }
              frame True {
                n710 = call "PCO_CloseCamera.vi"("ph"=w768) -> ()  [unwired: 9 in, 2 out]
              }
            }
          }
        }
        frame #2 {
          n711 = Array Size(array=w770) -> (size(s)=w771:i32)
          n712 = Initialize Array(u32 0 ("element"), w771) -> (w769:u32[])
          n713 = local write "phCam"(w769) -> ()
        }
      }
    }
  }
  n714 = Stop(stop? (T)=w1) -> ()
